vi "Main Responder.vi"(11 "CIFPluginManager in":refnum<class "CIFPluginManager.lvclass">) -> (0 "error out":errorcluster, 3 "Plugin Manager out":refnum<class "CIFPluginManager.lvclass">)   [LabVIEW 2021, in "CIFPluginManager.lvclass"]
uses:
  CIFPluginManager.lvclass
  gRPC/CIF_Manager_server/RPC Messages/cif_manager_RegisterPluginResponse.ctl
  CIFPluginManager.lvclass/CIFPluginManager.ctl
  <vilib>/Utility/miscctls.llb/LVMapReplaceAction.ctl
  gRPC/CIF_Manager_server/RPC Messages/cif_common_Empty.ctl
  <vilib>/CIF Foundation/CIF Core/CIFUtilities/CIFLogs/Typedef/Message Type.ctl
  <vilib>/CIF Foundation/CIF Core/CIFPluginManager/gRPC/CIF_Manager_client/RPC Messages/cif_common_Empty.ctl
  gRPC/CIF_Manager_server/RPC Messages/cif_manager_UnregisterPluginLoaderResponse.ctl
  gRPC/CIF_Manager_server/RPC Messages/cif_manager_QueryPluginTypesResponse.ctl
  gRPC/CIF_Manager_server/RPC Messages/cif_manager_PluginType.ctl
  gRPC/CIF_Manager_server/RPC Messages/cif_common_ShortVersion.ctl
  gRPC/CIF_Manager_server/RPC Messages/cif_management_common_PluginMetadata.ctl
  gRPC/CIF_Manager_server/RPC Messages/cif_manager_QueryAllChannelsResponse.ctl
  gRPC/CIF_Manager_server/RPC Messages/cif_management_common_Channels.ctl
  gRPC/CIF_Manager_server/RPC Messages/cif_management_common_Channel.ctl
  gRPC/CIF_Manager_server/RPC Messages/cif_management_common_ChannelDirection.ctl
  gRPC/CIF_Manager_server/RPC Messages/cif_management_common_ChannelPattern.ctl
  gRPC/CIF_Manager_server/RPC Messages/cif_manager_PingResponse.ctl
  gRPC/CIF_Manager_server/RPC Messages/cif_common_Status.ctl
  gRPC/CIF_Manager_server/RPC Messages/cif_manager_QueryErrorsResponse.ctl
  gRPC/CIF_Manager_server/RPC Messages/cif_manager_ErrorInfoList.ctl
  gRPC/CIF_Manager_server/RPC Messages/cif_manager_ErrorInfo.ctl
  gRPC/CIF_Manager_server/RPC Messages/cif_manager_QueryConfigResponse.ctl
  gRPC/CIF_Manager_server/RPC Messages/cif_manager_FileData.ctl
  gRPC/CIF_Manager_server/RPC Messages/cif_manager_QueryInfoResponse.ctl
  gRPC/CIF_Manager_server/RPC Messages/cif_manager_ResetErrorIndexResponse.ctl
  gRPC/CIF_Manager_server/RPC Messages/cif_manager_ResetConfigIndexResponse.ctl
  gRPC/CIF_Manager_server/RPC Messages/cif_manager_ResetInfoIndexResponse.ctl
  gRPC/CIF_Manager_server/RPC Messages/cif_manager_QueryPluginInfoResponse.ctl
  gRPC/CIF_Manager_server/RPC Messages/cif_manager_PluginInfoArray.ctl
  gRPC/CIF_Manager_server/RPC Messages/cif_manager_PluginInfo.ctl
  gRPC/CIF_Manager_server/RPC Messages/cif_management_common_PluginStatusData.ctl
  gRPC/CIF_Manager_server/RPC Messages/cif_management_common_PluginStatusData_PluginState.ctl
  gRPC/CIF_Manager_server/RPC Messages/cif_management_common_TimingStatistics.ctl
  gRPC/CIF_Manager_server/RPC Messages/cif_common_TimingStats.ctl
  gRPC/CIF_Manager_server/RPC Messages/cif_management_common_FifoStatistics.ctl
  gRPC/CIF_Manager_server/RPC Messages/cif_management_common_Error.ctl
  gRPC/CIF_Manager_server/RPC Messages/cif_management_common_MonitorDoubles.ctl
  gRPC/CIF_Manager_server/RPC Messages/cif_management_common_MonitorU64.ctl
  gRPC/CIF_Manager_server/RPC Messages/cif_management_common_MonitorI64.ctl
  gRPC/CIF_Manager_server/RPC Messages/cif_management_common_LoaderInfo.ctl
  gRPC/CIF_Manager_server/RPC Messages/cif_management_common_LoaderType.ctl
  gRPC/CIF_Manager_server/RPC Messages/cif_manager_QueryPluginResponse.ctl
  <vilib>/CIF Foundation/CIF Core/CIFCore/Common/Typedef/Errors.ctl
  gRPC/CIF_Manager_server/RPC Messages/cif_manager_QueryClockStatusResponse.ctl
  gRPC/CIF_Manager_server/RPC Messages/cif_manager_ClockStatusArray.ctl
  gRPC/CIF_Manager_server/RPC Messages/cif_manager_ClockStatus.ctl
  gRPC/CIF_Manager_server/RPC Messages/cif_manager_ClockConversion.ctl
  gRPC/CIF_Manager_server/RPC Messages/cif_manager_TimePair.ctl
  gRPC/CIF_Manager_server/RPC Messages/cif_manager_UpdateClockResponse.ctl
  <vilib>/CIF Foundation/CIF Utilities/Time/Typedef/Timestamp Pair.ctl
  gRPC/CIF_Manager_server/RPC Messages/cif_manager_CreateOrchResponse.ctl
  gRPC/CIF_Manager_server/RPC Messages/cif_manager_DestroyPluginLoaderResponse.ctl
  gRPC/CIF_Manager_server/RPC Messages/Get cif_manager_RegisterPluginRequest.vi
  gRPC/CIF_Manager_server/RPC Messages/Set cif_manager_RegisterPluginResponse.vi
  gRPC/CIF_Manager_server/RPC Messages/Get cif_manager_RegisterPluginLoaderRequest.vi
  gRPC/CIF_Manager_server/RPC Messages/Set cif_manager_RegisterPluginLoaderResponse.vi
  gRPC/CIF_Manager_server/RPC Messages/Get cif_manager_UnregisterPluginRequest.vi
  gRPC/CIF_Manager_server/RPC Messages/Set cif_manager_UnregisterPluginResponse.vi
  gRPC/CIF_Manager_server/RPC Messages/Get cif_manager_UnregisterPluginLoaderRequest.vi
  gRPC/CIF_Manager_server/RPC Messages/Set cif_manager_UnregisterPluginLoaderResponse.vi
  gRPC/CIF_Manager_server/RPC Messages/Get cif_manager_QueryPluginTypesRequest.vi
  gRPC/CIF_Manager_server/RPC Messages/Set cif_manager_QueryPluginTypesResponse.vi
  gRPC/CIF_Manager_server/RPC Messages/Get cif_manager_QueryAllChannelsRequest.vi
  gRPC/CIF_Manager_server/RPC Messages/Set cif_manager_QueryAllChannelsResponse.vi
  gRPC/CIF_Manager_server/RPC Messages/Get cif_manager_DestroyRequest.vi
  gRPC/CIF_Manager_server/RPC Messages/Set cif_manager_DestroyResponse.vi
  gRPC/CIF_Manager_server/RPC Messages/Get cif_manager_PingRequest.vi
  gRPC/CIF_Manager_server/RPC Messages/Set cif_manager_PingResponse.vi
  gRPC/CIF_Manager_server/RPC Messages/Get cif_manager_QueryErrorsRequest.vi
  gRPC/CIF_Manager_server/RPC Messages/Set cif_manager_QueryErrorsResponse.vi
  gRPC/CIF_Manager_server/RPC Messages/Get cif_manager_QueryConfigRequest.vi
  gRPC/CIF_Manager_server/RPC Messages/Set cif_manager_QueryConfigResponse.vi
  gRPC/CIF_Manager_server/RPC Messages/Get cif_manager_QueryInfoRequest.vi
  gRPC/CIF_Manager_server/RPC Messages/Set cif_manager_QueryInfoResponse.vi
  gRPC/CIF_Manager_server/RPC Messages/Get cif_manager_ResetErrorIndexRequest.vi
  gRPC/CIF_Manager_server/RPC Messages/Set cif_manager_ResetErrorIndexResponse.vi
  gRPC/CIF_Manager_server/RPC Messages/Get cif_manager_ResetConfigIndexRequest.vi
  gRPC/CIF_Manager_server/RPC Messages/Set cif_manager_ResetConfigIndexResponse.vi
  gRPC/CIF_Manager_server/RPC Messages/Get cif_manager_ResetInfoIndexRequest.vi
  gRPC/CIF_Manager_server/RPC Messages/Set cif_manager_ResetInfoIndexResponse.vi
  gRPC/CIF_Manager_server/RPC Messages/Get cif_manager_QueryPluginInfoRequest.vi
  gRPC/CIF_Manager_server/RPC Messages/Set cif_manager_QueryPluginInfoResponse.vi
  gRPC/CIF_Manager_server/RPC Messages/Get cif_manager_QueryPluginRequest.vi
  gRPC/CIF_Manager_server/RPC Messages/Set cif_manager_QueryPluginResponse.vi
  <vilib>/CIF Foundation/CIF Utilities/Errors/Append Error Location.vi
  gRPC/CIF_Manager_server/RPC Messages/Get cif_manager_QueryClockStatusRequest.vi
  gRPC/CIF_Manager_server/RPC Messages/Set cif_manager_QueryClockStatusResponse.vi
  gRPC/CIF_Manager_server/RPC Messages/Get cif_manager_UpdateClockRequest.vi
  gRPC/CIF_Manager_server/RPC Messages/Set cif_manager_UpdateClockResponse.vi
  <vilib>/CIF Foundation/CIF Utilities/Time/SubVIs/Weighted Moving Average for Slope.vi
  <vilib>/CIF Foundation/CIF Utilities/DataTypes/Utilities/Valid Number.vi
  gRPC/CIF_Manager_server/RPC Messages/Get cif_manager_CreateOrchRequest.vi
  gRPC/CIF_Manager_server/RPC Messages/Set cif_manager_CreateOrchResponse.vi
  gRPC/CIF_Manager_server/RPC Messages/Get cif_manager_DestroyPluginLoaderRequest.vi
  gRPC/CIF_Manager_server/RPC Messages/Set cif_manager_DestroyPluginLoaderResponse.vi
  gRPC/CIF_Manager_server/RPC Messages/Get cif_manager_RegisterPluginRequest.vi/2ed25e12-861d-4677-8ead-ace2906b2041.vi
  gRPC/CIF_Manager_server/RPC Messages/FlatToRichcif_manager_RegisterPluginRequest.vi
  gRPC/CIF_Manager_server/RPC Messages/Set cif_manager_RegisterPluginResponse.vi/dcc74a39-081a-4bdd-860b-8ed792803c96.vi
  gRPC/CIF_Manager_server/RPC Messages/RichToFlatcif_manager_RegisterPluginResponse.vi
  gRPC/CIF_Manager_server/RPC Messages/Get cif_manager_RegisterPluginLoaderRequest.vi/2ed25e12-861d-4677-8ead-ace2906b2041.vi
  gRPC/CIF_Manager_server/RPC Messages/FlatToRichcif_manager_RegisterPluginLoaderRequest.vi
  gRPC/CIF_Manager_server/RPC Messages/Set cif_manager_RegisterPluginLoaderResponse.vi/dcc74a39-081a-4bdd-860b-8ed792803c96.vi
  gRPC/CIF_Manager_server/RPC Messages/RichToFlatcif_manager_RegisterPluginLoaderResponse.vi
  gRPC/CIF_Manager_server/RPC Messages/Get cif_manager_UnregisterPluginRequest.vi/2ed25e12-861d-4677-8ead-ace2906b2041.vi
  gRPC/CIF_Manager_server/RPC Messages/FlatToRichcif_manager_UnregisterPluginRequest.vi
  gRPC/CIF_Manager_server/RPC Messages/Set cif_manager_UnregisterPluginResponse.vi/dcc74a39-081a-4bdd-860b-8ed792803c96.vi
  gRPC/CIF_Manager_server/RPC Messages/RichToFlatcif_manager_UnregisterPluginResponse.vi
  gRPC/CIF_Manager_server/RPC Messages/Get cif_manager_UnregisterPluginLoaderRequest.vi/2ed25e12-861d-4677-8ead-ace2906b2041.vi
  gRPC/CIF_Manager_server/RPC Messages/FlatToRichcif_manager_UnregisterPluginLoaderRequest.vi
  gRPC/CIF_Manager_server/RPC Messages/Set cif_manager_UnregisterPluginLoaderResponse.vi/dcc74a39-081a-4bdd-860b-8ed792803c96.vi
  gRPC/CIF_Manager_server/RPC Messages/RichToFlatcif_manager_UnregisterPluginLoaderResponse.vi
  gRPC/CIF_Manager_server/RPC Messages/Get cif_manager_QueryPluginTypesRequest.vi/2ed25e12-861d-4677-8ead-ace2906b2041.vi
  gRPC/CIF_Manager_server/RPC Messages/FlatToRichcif_manager_QueryPluginTypesRequest.vi
  gRPC/CIF_Manager_server/RPC Messages/Set cif_manager_QueryPluginTypesResponse.vi/dcc74a39-081a-4bdd-860b-8ed792803c96.vi
  gRPC/CIF_Manager_server/RPC Messages/RichToFlatcif_manager_QueryPluginTypesResponse.vi
  gRPC/CIF_Manager_server/RPC Messages/Get cif_manager_QueryAllChannelsRequest.vi/2ed25e12-861d-4677-8ead-ace2906b2041.vi
  gRPC/CIF_Manager_server/RPC Messages/FlatToRichcif_manager_QueryAllChannelsRequest.vi
  gRPC/CIF_Manager_server/RPC Messages/Set cif_manager_QueryAllChannelsResponse.vi/dcc74a39-081a-4bdd-860b-8ed792803c96.vi
  gRPC/CIF_Manager_server/RPC Messages/RichToFlatcif_manager_QueryAllChannelsResponse.vi
  gRPC/CIF_Manager_server/RPC Messages/Get cif_manager_DestroyRequest.vi/2ed25e12-861d-4677-8ead-ace2906b2041.vi
  gRPC/CIF_Manager_server/RPC Messages/FlatToRichcif_manager_DestroyRequest.vi
  gRPC/CIF_Manager_server/RPC Messages/Set cif_manager_DestroyResponse.vi/dcc74a39-081a-4bdd-860b-8ed792803c96.vi
  gRPC/CIF_Manager_server/RPC Messages/RichToFlatcif_manager_DestroyResponse.vi
  gRPC/CIF_Manager_server/RPC Messages/Get cif_manager_PingRequest.vi/2ed25e12-861d-4677-8ead-ace2906b2041.vi
  gRPC/CIF_Manager_server/RPC Messages/FlatToRichcif_manager_PingRequest.vi
  gRPC/CIF_Manager_server/RPC Messages/Set cif_manager_PingResponse.vi/dcc74a39-081a-4bdd-860b-8ed792803c96.vi
  gRPC/CIF_Manager_server/RPC Messages/RichToFlatcif_manager_PingResponse.vi
  gRPC/CIF_Manager_server/RPC Messages/Get cif_manager_QueryErrorsRequest.vi/2ed25e12-861d-4677-8ead-ace2906b2041.vi
  gRPC/CIF_Manager_server/RPC Messages/FlatToRichcif_manager_QueryErrorsRequest.vi
  gRPC/CIF_Manager_server/RPC Messages/Set cif_manager_QueryErrorsResponse.vi/dcc74a39-081a-4bdd-860b-8ed792803c96.vi
  gRPC/CIF_Manager_server/RPC Messages/RichToFlatcif_manager_QueryErrorsResponse.vi
  gRPC/CIF_Manager_server/RPC Messages/Get cif_manager_QueryConfigRequest.vi/2ed25e12-861d-4677-8ead-ace2906b2041.vi
  gRPC/CIF_Manager_server/RPC Messages/FlatToRichcif_manager_QueryConfigRequest.vi
  gRPC/CIF_Manager_server/RPC Messages/Set cif_manager_QueryConfigResponse.vi/dcc74a39-081a-4bdd-860b-8ed792803c96.vi
  gRPC/CIF_Manager_server/RPC Messages/RichToFlatcif_manager_QueryConfigResponse.vi
  gRPC/CIF_Manager_server/RPC Messages/Get cif_manager_QueryInfoRequest.vi/2ed25e12-861d-4677-8ead-ace2906b2041.vi
  gRPC/CIF_Manager_server/RPC Messages/FlatToRichcif_manager_QueryInfoRequest.vi
  gRPC/CIF_Manager_server/RPC Messages/Set cif_manager_QueryInfoResponse.vi/dcc74a39-081a-4bdd-860b-8ed792803c96.vi
  gRPC/CIF_Manager_server/RPC Messages/RichToFlatcif_manager_QueryInfoResponse.vi
  gRPC/CIF_Manager_server/RPC Messages/Get cif_manager_ResetErrorIndexRequest.vi/2ed25e12-861d-4677-8ead-ace2906b2041.vi
  gRPC/CIF_Manager_server/RPC Messages/FlatToRichcif_manager_ResetErrorIndexRequest.vi
  gRPC/CIF_Manager_server/RPC Messages/Set cif_manager_ResetErrorIndexResponse.vi/dcc74a39-081a-4bdd-860b-8ed792803c96.vi
  gRPC/CIF_Manager_server/RPC Messages/RichToFlatcif_manager_ResetErrorIndexResponse.vi
  gRPC/CIF_Manager_server/RPC Messages/Get cif_manager_ResetConfigIndexRequest.vi/2ed25e12-861d-4677-8ead-ace2906b2041.vi
  gRPC/CIF_Manager_server/RPC Messages/FlatToRichcif_manager_ResetConfigIndexRequest.vi
  gRPC/CIF_Manager_server/RPC Messages/Set cif_manager_ResetConfigIndexResponse.vi/dcc74a39-081a-4bdd-860b-8ed792803c96.vi
  gRPC/CIF_Manager_server/RPC Messages/RichToFlatcif_manager_ResetConfigIndexResponse.vi
  gRPC/CIF_Manager_server/RPC Messages/Get cif_manager_ResetInfoIndexRequest.vi/2ed25e12-861d-4677-8ead-ace2906b2041.vi
  gRPC/CIF_Manager_server/RPC Messages/FlatToRichcif_manager_ResetInfoIndexRequest.vi
  gRPC/CIF_Manager_server/RPC Messages/Set cif_manager_ResetInfoIndexResponse.vi/dcc74a39-081a-4bdd-860b-8ed792803c96.vi
  gRPC/CIF_Manager_server/RPC Messages/RichToFlatcif_manager_ResetInfoIndexResponse.vi
  gRPC/CIF_Manager_server/RPC Messages/Get cif_manager_QueryPluginInfoRequest.vi/2ed25e12-861d-4677-8ead-ace2906b2041.vi
  gRPC/CIF_Manager_server/RPC Messages/FlatToRichcif_manager_QueryPluginInfoRequest.vi
  gRPC/CIF_Manager_server/RPC Messages/Set cif_manager_QueryPluginInfoResponse.vi/dcc74a39-081a-4bdd-860b-8ed792803c96.vi
  gRPC/CIF_Manager_server/RPC Messages/RichToFlatcif_manager_QueryPluginInfoResponse.vi
  gRPC/CIF_Manager_server/RPC Messages/Get cif_manager_QueryPluginRequest.vi/2ed25e12-861d-4677-8ead-ace2906b2041.vi
  gRPC/CIF_Manager_server/RPC Messages/FlatToRichcif_manager_QueryPluginRequest.vi
  gRPC/CIF_Manager_server/RPC Messages/Set cif_manager_QueryPluginResponse.vi/dcc74a39-081a-4bdd-860b-8ed792803c96.vi
  gRPC/CIF_Manager_server/RPC Messages/RichToFlatcif_manager_QueryPluginResponse.vi
  gRPC/CIF_Manager_server/RPC Messages/Get cif_manager_QueryClockStatusRequest.vi/2ed25e12-861d-4677-8ead-ace2906b2041.vi
  gRPC/CIF_Manager_server/RPC Messages/FlatToRichcif_manager_QueryClockStatusRequest.vi
  gRPC/CIF_Manager_server/RPC Messages/Set cif_manager_QueryClockStatusResponse.vi/dcc74a39-081a-4bdd-860b-8ed792803c96.vi
  gRPC/CIF_Manager_server/RPC Messages/RichToFlatcif_manager_QueryClockStatusResponse.vi
  gRPC/CIF_Manager_server/RPC Messages/Get cif_manager_UpdateClockRequest.vi/2ed25e12-861d-4677-8ead-ace2906b2041.vi
  gRPC/CIF_Manager_server/RPC Messages/FlatToRichcif_manager_UpdateClockRequest.vi
  gRPC/CIF_Manager_server/RPC Messages/Set cif_manager_UpdateClockResponse.vi/dcc74a39-081a-4bdd-860b-8ed792803c96.vi
  gRPC/CIF_Manager_server/RPC Messages/RichToFlatcif_manager_UpdateClockResponse.vi
  <vilib>/Analysis/3filter.llb/Savitzky-Golay Filter.vi
  <vilib>/Analysis/3filter.llb/Savitzky-Golay Filter (DBL).vi
  gRPC/CIF_Manager_server/RPC Messages/Get cif_manager_CreateOrchRequest.vi/2ed25e12-861d-4677-8ead-ace2906b2041.vi
  gRPC/CIF_Manager_server/RPC Messages/FlatToRichcif_manager_CreateOrchRequest.vi
  gRPC/CIF_Manager_server/RPC Messages/Set cif_manager_CreateOrchResponse.vi/dcc74a39-081a-4bdd-860b-8ed792803c96.vi
  gRPC/CIF_Manager_server/RPC Messages/RichToFlatcif_manager_CreateOrchResponse.vi
  gRPC/CIF_Manager_server/RPC Messages/Get cif_manager_DestroyPluginLoaderRequest.vi/2ed25e12-861d-4677-8ead-ace2906b2041.vi
  gRPC/CIF_Manager_server/RPC Messages/FlatToRichcif_manager_DestroyPluginLoaderRequest.vi
  gRPC/CIF_Manager_server/RPC Messages/Set cif_manager_DestroyPluginLoaderResponse.vi/dcc74a39-081a-4bdd-860b-8ed792803c96.vi
  gRPC/CIF_Manager_server/RPC Messages/RichToFlatcif_manager_DestroyPluginLoaderResponse.vi
  <vilib>/gRPC/LabVIEW gRPC Library/Shared/TranslateGrpcError.vi
  gRPC/CIF_Manager_server/RPC Messages/FlatToRichcif_common_ShortVersion.vi
  gRPC/CIF_Manager_server/RPC Messages/FlatToRichcif_management_common_LoaderInfoFull.vi
  gRPC/CIF_Manager_server/RPC Messages/RichToFlatcif_manager_PluginType.vi
  gRPC/CIF_Manager_server/RPC Messages/FlatToRichcif_management_common_ChannelFilter.vi
  gRPC/CIF_Manager_server/RPC Messages/RichToFlatcif_management_common_Channels.vi
  gRPC/CIF_Manager_server/RPC Messages/RichToFlatcif_common_Status.vi
  gRPC/CIF_Manager_server/RPC Messages/FlatToRichcif_manager_QuerySettings.vi
  gRPC/CIF_Manager_server/RPC Messages/RichToFlatcif_manager_ErrorInfoList.vi
  gRPC/CIF_Manager_server/RPC Messages/RichToFlatcif_manager_FileData.vi
  gRPC/CIF_Manager_server/RPC Messages/RichToFlatcif_manager_PluginInfoArray.vi
  gRPC/CIF_Manager_server/RPC Messages/RichToFlatcif_manager_PluginInfo.vi
  gRPC/CIF_Manager_server/RPC Messages/RichToFlatcif_manager_ClockStatusArray.vi
  gRPC/CIF_Manager_server/RPC Messages/FlatToRichcif_manager_TimePair.vi
  gRPC/CIF_Manager_server/RPC Messages/RichToFlatcif_common_ShortVersion.vi
  gRPC/CIF_Manager_server/RPC Messages/RichToFlatcif_management_common_PluginMetadata.vi
  gRPC/CIF_Manager_server/RPC Messages/RichToFlatcif_management_common_Channel.vi
  gRPC/CIF_Manager_server/RPC Messages/RichToFlatcif_manager_ErrorInfo.vi
  gRPC/CIF_Manager_server/RPC Messages/RichToFlatcif_management_common_PluginStatusData.vi
  gRPC/CIF_Manager_server/RPC Messages/RichToFlatcif_management_common_LoaderInfo.vi
  gRPC/CIF_Manager_server/RPC Messages/RichToFlatcif_manager_ClockStatus.vi
  gRPC/CIF_Manager_server/RPC Messages/RichToFlatcif_management_common_TimingStatistics.vi
  gRPC/CIF_Manager_server/RPC Messages/RichToFlatcif_management_common_FifoStatistics.vi
  gRPC/CIF_Manager_server/RPC Messages/RichToFlatcif_management_common_Error.vi
  gRPC/CIF_Manager_server/RPC Messages/RichToFlatcif_management_common_MonitorDoubles.vi
  gRPC/CIF_Manager_server/RPC Messages/RichToFlatcif_management_common_MonitorU64.vi
  gRPC/CIF_Manager_server/RPC Messages/RichToFlatcif_management_common_MonitorI64.vi
  gRPC/CIF_Manager_server/RPC Messages/RichToFlatcif_manager_ClockConversion.vi
  gRPC/CIF_Manager_server/RPC Messages/RichToFlatcif_common_TimingStats.vi
  gRPC/CIF_Manager_server/RPC Messages/RichToFlatcif_manager_TimePair.vi
  <vilib>/gRPC/LabVIEW gRPC Library/Server API/Server/Get Server DLL Path.vi
  <vilib>/Utility/error.llb/Error Cluster From Error Code.vi
  <vilib>/gRPC/LabVIEW gRPC Library/Server API/Message Requests/Complete Call.vi
  <vilib>/Analysis/baseanly.llb/Std Deviation and Variance.vi
  <vilib>/Analysis/6fits.llb/Linear Fit.vi
  <vilib>/regexp/Match Regular Expression.xnode
  <vilib>/CIF Foundation/CIF Core/CIFUtilities/CIFLogs/CIFLogs.lvlib
  <vilib>/CIF Foundation/CIF Core/CIFPluginManager/gRPC/CIF_Manager_Client_Wrapper/CIFManagerClientWrapper.lvlib
  <vilib>/CIF Foundation/CIF Core/CIFPluginManager/gRPC/CIF_Manager_client/CIF_Manager_client.lvlib
  gRPC/CIF_Manager_server/RPC Service/Manager/Manager.lvclass
  <vilib>/CIF Foundation/CIF Utilities/Time/Time_CIF_U.lvlib
  <vilib>/CIF Foundation/CIF Core/CIFCore/Grpc/CIFCoreWrapper/CIFCoreWrapper.lvlib
  <vilib>/CIF Foundation/CIF Core/CIFUtilities/CIFConfigurationFile/CIF Configuration File.lvlib
  gRPC/CIF_Manager_server/CIF_Manager_server.lvlib
  CIFPluginLoader/gRPC/CIF_Plugin_Loader_Client_Wrapper/CIFPluginLoaderClientWrapper.lvlib
  <vilib>/CIF Foundation/CIF Core/CIFCore/Common/CIFCoreCommon.lvlib
  CIFUtilities/Scripting/Orchestration/Python/Python Orchestration.lvlib
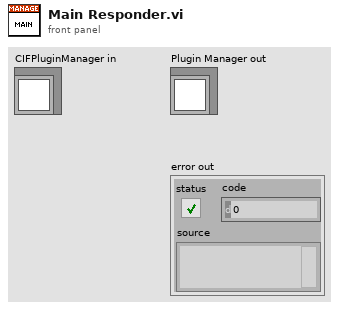
[diagram p1: front panel]
types:
  T1 = typedef "CIF_Manager_server.lvlib/cif_manager_RegisterPluginResponse.ctl" = cluster{"loader_name":string}
  T2 = typedef "LVMapReplaceAction.ctl" = enum32{"Modify Entry only if found", "Add or Modify Entry", "Delete Entry"}
  T3 = typedef "CIF_Manager_server.lvlib/cif_common_Empty.ctl" = cluster{"void":string}
  T4 = typedef "CIFLogs.lvlib/Message Type.ctl" = enum16{"Error", "Information", "Print Terminal", "Configuration"}
  T5 = typedef "CIF_Manager_client.lvlib/cif_common_Empty.ctl" = cluster{"void":string}
  T6 = typedef "CIF_Manager_server.lvlib/cif_manager_UnregisterPluginLoaderResponse.ctl" = cluster{"void":string}
  T7 = typedef "CIF_Manager_server.lvlib/cif_manager_QueryPluginTypesResponse.ctl" = cluster{"plugin_types":T8[]}
  T8 = typedef "CIF_Manager_server.lvlib/cif_manager_PluginType.ctl" = cluster{"plugin_type":string, "plugin_version":T9, "plugin_metadata":T10, "relative_path":string[]}
  T9 = typedef "CIF_Manager_server.lvlib/cif_common_ShortVersion.ctl" = cluster{"major":u32, "minor":u32, "fix":u32}
  T10 = typedef "CIF_Manager_server.lvlib/cif_management_common_PluginMetadata.ctl" = cluster{"description":string, "history":string, "author":string}
  T11 = typedef "CIF_Manager_server.lvlib/cif_manager_QueryAllChannelsResponse.ctl" = cluster{"channels":T12}
  T12 = typedef "CIF_Manager_server.lvlib/cif_management_common_Channels.ctl" = cluster{"channels":T13[]}
  T13 = typedef "CIF_Manager_server.lvlib/cif_management_common_Channel.ctl" = cluster{"name":string, "direction":T14, "type":string, "custom_config":u8[], "connected":bool, "connected_name":string, "forced":bool, "channel_pattern":T15}
  T14 = typedef "CIF_Manager_server.lvlib/cif_management_common_ChannelDirection.ctl" = enum32{"CHANNELDIRECTION_UNKNOWN", "CHANNELDIRECTION_PUBLISHER", "CHANNELDIRECTION_SUBSCRIBER"}
  T15 = typedef "CIF_Manager_server.lvlib/cif_management_common_ChannelPattern.ctl" = enum32{"CHANNELPATTERN_UNKNOWN", "CHANNELPATTERN_TAG", "CHANNELPATTERN_FIFO", "CHANNELPATTERN_MULTIFIFO", "CHANNELPATTERN_BACKPRESSUREFIFO"}
  T16 = typedef "CIF_Manager_server.lvlib/cif_manager_PingResponse.ctl" = cluster{"status":T17}
  T17 = typedef "CIF_Manager_server.lvlib/cif_common_Status.ctl" = cluster{"code":i32, "message":string}
  T18 = typedef "CIF_Manager_server.lvlib/cif_manager_QueryErrorsResponse.ctl" = cluster{"error_info_list":T19}
  T19 = typedef "CIF_Manager_server.lvlib/cif_manager_ErrorInfoList.ctl" = cluster{"error_info":T20[]}
  T20 = typedef "CIF_Manager_server.lvlib/cif_manager_ErrorInfo.ctl" = cluster{"error_status":bool, "error_code":i32, "plugin":string, "time":string, "message":string, "location":string}
  T21 = typedef "CIF_Manager_server.lvlib/cif_manager_QueryConfigResponse.ctl" = cluster{"file_data":T22}
  T22 = typedef "CIF_Manager_server.lvlib/cif_manager_FileData.ctl" = cluster{"data":string}
  T23 = typedef "CIF_Manager_server.lvlib/cif_manager_QueryInfoResponse.ctl" = cluster{"file_data":T22}
  T24 = typedef "CIF_Manager_server.lvlib/cif_manager_ResetErrorIndexResponse.ctl" = cluster{"status":T17}
  T25 = typedef "CIF_Manager_server.lvlib/cif_manager_ResetConfigIndexResponse.ctl" = cluster{"status":T17}
  T26 = typedef "CIF_Manager_server.lvlib/cif_manager_ResetInfoIndexResponse.ctl" = cluster{"status":T17}
  T27 = typedef "CIF_Manager_server.lvlib/cif_manager_QueryPluginInfoResponse.ctl" = cluster{"plugin_info_array":T28}
  T28 = typedef "CIF_Manager_server.lvlib/cif_manager_PluginInfoArray.ctl" = cluster{"plugin_info":T29[]}
  T29 = typedef "CIF_Manager_server.lvlib/cif_manager_PluginInfo.ctl" = cluster{"plugin_name":string, "plugin_type":string, "grpc_port":i32, "plugin_version":T9, "status":T30, "loader_info":T39}
  T30 = typedef "CIF_Manager_server.lvlib/cif_management_common_PluginStatusData.ctl" = cluster{"state":T31, "timing_statistics":T32, "fifo_statistics":T34, "error":T35, "monitor_doubles":T36, "monitor_u64s":T37, "monitor_i64s":T38}
  T31 = typedef "CIF_Manager_server.lvlib/cif_management_common_PluginStatusData_PluginState.ctl" = enum32{"PLUGINSTATE_UNKNOWN", "PLUGINSTATE_CREATING", "PLUGINSTATE_LISTENING", "PLUGINSTATE_RUNNING", "PLUGINSTATE_CLEANINGUP", "PLUGINSTATE_DESTROYING"}
  T32 = typedef "CIF_Manager_server.lvlib/cif_management_common_TimingStatistics.ctl" = cluster{"period":T33, "wake_error":T33, "execute":T33, "housekeep":T33, "idle":T33, "cleanup":T33, "custom_1":T33, "custom_2":T33}
  T33 = typedef "CIF_Manager_server.lvlib/cif_common_TimingStats.ctl" = cluster{"max":i64, "min":i64, "avg":dbl}
  T34 = typedef "CIF_Manager_server.lvlib/cif_management_common_FifoStatistics.ctl" = cluster{"from_t0":T33, "from_previous_plugin":T33, "output_error":T33}
  T35 = typedef "CIF_Manager_server.lvlib/cif_management_common_Error.ctl" = cluster{"status":bool, "code":i32}
  T36 = typedef "CIF_Manager_server.lvlib/cif_management_common_MonitorDoubles.ctl" = cluster{"double_1":dbl, "double_2":dbl, "double_3":dbl, "double_4":dbl}
  T37 = typedef "CIF_Manager_server.lvlib/cif_management_common_MonitorU64.ctl" = cluster{"u64_1":u64, "u64_2":u64, "u64_3":u64, "u64_4":u64}
  T38 = typedef "CIF_Manager_server.lvlib/cif_management_common_MonitorI64.ctl" = cluster{"i64_1":i64, "i64_2":i64, "i64_3":i64, "i64_4":i64}
  T39 = typedef "CIF_Manager_server.lvlib/cif_management_common_LoaderInfo.ctl" = cluster{"loader_type":T40, "loader_name":string}
  T40 = typedef "CIF_Manager_server.lvlib/cif_management_common_LoaderType.ctl" = enum32{"LOADERTYPE_UNKNOWN", "LOADERTYPE_LABVIEW"}
  T41 = typedef "CIF_Manager_server.lvlib/cif_manager_QueryPluginResponse.ctl" = cluster{"plugin_info":T29, "status":T17}
  T42 = typedef "CIFCoreCommon.lvlib/Errors.ctl" = enum16{"Invalid Clock ID", "Long Sleep", "gRPC Server Not Found", "Config Parse", "Timestamp Wrap", "Delayed Execution", "Duplicate Channel", "Missing Channel", "Incorrect Type", "Flatten Error", "Unflatten Data", "Unique Name", "Plugin Not Found", "Plugin Type Not Found", "Plugin Version Not Found", "Manager Not Found", "Numerical Issue", "Time Jump", "Clock ID Match", "Channel Length", "Plugin Connection", "gRPC Server Connection", "PPL Name Match", "Build", "Config Log Parse", "Plugin Load", "UI Subpanel Load", "Python Name", "Invalid Name", "Unable to Change Ch Buffer", "Failed Kill", "Failed SysExec", "Function Not Implemented", "Load Timeout"}
  T43 = typedef "CIF_Manager_server.lvlib/cif_manager_QueryClockStatusResponse.ctl" = cluster{"clock_status_array":T44}
  T44 = typedef "CIF_Manager_server.lvlib/cif_manager_ClockStatusArray.ctl" = cluster{"clocks_status":T45[]}
  T45 = typedef "CIF_Manager_server.lvlib/cif_manager_ClockStatus.ctl" = cluster{"clock_conversion":T46, "error_mean":i64, "error_std_dev":i64}
  T46 = typedef "CIF_Manager_server.lvlib/cif_manager_ClockConversion.ctl" = cluster{"clock_id":u32, "last_reset":i64, "slope":dbl, "offset_pair":T47, "clock_name":string}
  T47 = typedef "CIF_Manager_server.lvlib/cif_manager_TimePair.ctl" = cluster{"system_time":i64, "external_time":i64}
  T48 = typedef "CIF_Manager_server.lvlib/cif_manager_UpdateClockResponse.ctl" = cluster{"status":T17}
  T49 = typedef "Time_CIF_U.lvlib/Timestamp Pair.ctl" = cluster{"System Time":i64, "External Time":i64}
  T50 = typedef "CIF_Manager_server.lvlib/cif_manager_CreateOrchResponse.ctl" = cluster{"orchestration_script":string, "status":T17}
  T51 = typedef "CIF_Manager_server.lvlib/cif_manager_DestroyPluginLoaderResponse.ctl" = cluster{"status":T17}
  T52 = typedef "grpc-lvsupport-release.lvlib/grpcId.ctl" = u64
  T53 = typedef "CIF_Manager_server.lvlib/cif_manager_RegisterPluginRequest.ctl" = cluster{"plugin_name":string, "grpc_port":i32, "plugin_version":T9}
  T54 = typedef "CIFPluginManager.lvclass/Plugin Management Data Map.ctl" = map{string, T55}
  T55 = typedef "CIFPluginManager.lvclass/Plugin Management Data.ctl" = cluster{"Unique Name":string, "Plugin Type":string, "gRPC Port":i32, "gRPC ID":T52, "Loader Type":T56, "Loader":string, "Version":T57, "Load Timestamp":i64, "Unload Timestamp":i64, "Unloading":bool, "Ready for removal":bool, "status":T30, "channels":T12}
  T56 = typedef "CIFPluginManager.lvclass/Loader Type.ctl" = enum16{"LabVIEW"}
  T57 = typedef "CIFCoreCommon.lvlib/Version.ctl" = cluster{"Major":i32, "Minor":i32, "Fix":i32, "Build":i32}
  T58 = typedef "CIF_Manager_server.lvlib/cif_manager_RegisterPluginLoaderRequest.ctl" = cluster{"loader_info":T59}
  T59 = typedef "CIF_Manager_server.lvlib/cif_management_common_LoaderInfoFull.ctl" = cluster{"loader_type":T40, "loader_name":string, "grpc_port":i32, "pid":u32}
  T60 = typedef "CIFPluginManager.lvclass/Loader Map.ctl" = map{string, T61}
  T61 = typedef "CIFPluginManager.lvclass/Loaders.ctl" = cluster{"Loader Type":T56, "grpc_port":i32, "pid":u32, "gRPC ID":T52, "Load Timestamp":i64, "Unloading":bool, "Ready for removal":bool, "Unload Timestamp":i64}
  T62 = typedef "CIF_Manager_server.lvlib/cif_manager_UnregisterPluginRequest.ctl" = cluster{"plugin_name":string, "unregister_channels":string[]}
  T63 = typedef "CIF_Manager_server.lvlib/cif_manager_UnregisterPluginLoaderRequest.ctl" = cluster{"loader_name":string}
  T64 = typedef "CIF_Manager_server.lvlib/cif_manager_QueryPluginTypesRequest.ctl" = cluster{"reload":bool}
  T65 = typedef "CIFPluginManager.lvclass/Discovered Plugin Map.ctl" = map{string, T66[]}
  T66 = typedef "CIFPluginManager.lvclass/Discovered Plugin.ctl" = cluster{"Filename":string, "Plugin Type":string, "Qualified name":string, "Version":T57, "Plugin Metadata":T67, "Loader Type":T56, "File Path":string, "Relative Path":string[]}
  T67 = typedef "CIFPluginManager.lvclass/Plugin Metadata.ctl" = cluster{"Description":string, "History":string, "Author":string}
  T68 = typedef "CIF_Manager_server.lvlib/cif_manager_QueryAllChannelsRequest.ctl" = cluster{"channel_filter":T69}
  T69 = typedef "CIF_Manager_server.lvlib/cif_management_common_ChannelFilter.ctl" = cluster{"name_regex":string, "direction":T14, "direction_filter":bool, "type_regex":string, "forced":bool, "forced_filter":bool}
  T70 = typedef "CIF_Manager_client.lvlib/cif_common_Status.ctl" = cluster{"code":i32, "message":string}
  T71 = typedef "CIF_Manager_server.lvlib/cif_manager_QueryErrorsRequest.ctl" = cluster{"query_settings":T72}
  T72 = typedef "CIF_Manager_server.lvlib/cif_manager_QuerySettings.ctl" = cluster{"query_all":bool}
  T73 = typedef "CIFLogs.lvlib/Error Message.ctl" = cluster{"error":bool, "code":i32, "Message":string, "Location":string, "Plugin":string, "Time":string}
  T74 = typedef "CIF_Manager_server.lvlib/cif_manager_QueryConfigRequest.ctl" = cluster{"query_settings":T72}
  T75 = typedef "CIF_Manager_server.lvlib/cif_manager_QueryInfoRequest.ctl" = cluster{"query_settings":T72}
  T76 = typedef "CIFLogs.lvlib/Log Info.ctl" = cluster{"size (bytes)":i64, "Last Timestamp":string}
  T77 = typedef "CIF_Manager_server.lvlib/cif_manager_QueryPluginRequest.ctl" = cluster{"plugin_name":string}
  T78 = typedef "Time_CIF_U.lvlib/Clock History Map.ctl" = map{u8, T79}
  T79 = typedef "Time_CIF_U.lvlib/Clock History.ctl" = cluster{"System Clock":i64[], "External Clock":i64[], "Last Reset Time":i64, "slope":dbl, "1/slope":dbl, "Offset Pair":T49, "Name":string}
  T80 = typedef "Time_CIF_U.lvlib/Clock Conversion.ctl" = cluster{"ClockID":u8, "Last Reset":i64, "Offset Pair":T49, "Slope":dbl, "1/Slope":dbl, "Name":string}
  T81 = typedef "Time_CIF_U.lvlib/Clock Error Statistics.ctl" = cluster{"mean":i64, "standard deviation":i64}
  T82 = typedef "CIF_Manager_server.lvlib/cif_manager_UpdateClockRequest.ctl" = cluster{"clock_id":u32, "timestamp_pair":T47, "reinit":bool, "clock_name":string}
  T83 = typedef "CIF_Manager_server.lvlib/cif_manager_CreateOrchRequest.ctl" = cluster{"start_timestamp":u64, "create_file":bool, "orchestration_language":T84, "filename":string, "default_ip":string}
  T84 = typedef "CIF_Manager_server.lvlib/cif_manager_OrchestrationLanguage.ctl" = enum32{"ORCHESTRATIONLANGUAGE_UNKNOWN", "ORCHESTRATIONLANGUAGE_PYTHON"}
  T85 = typedef "CIF_Manager_server.lvlib/cif_manager_DestroyPluginLoaderRequest.ctl" = cluster{"loader_name":string}
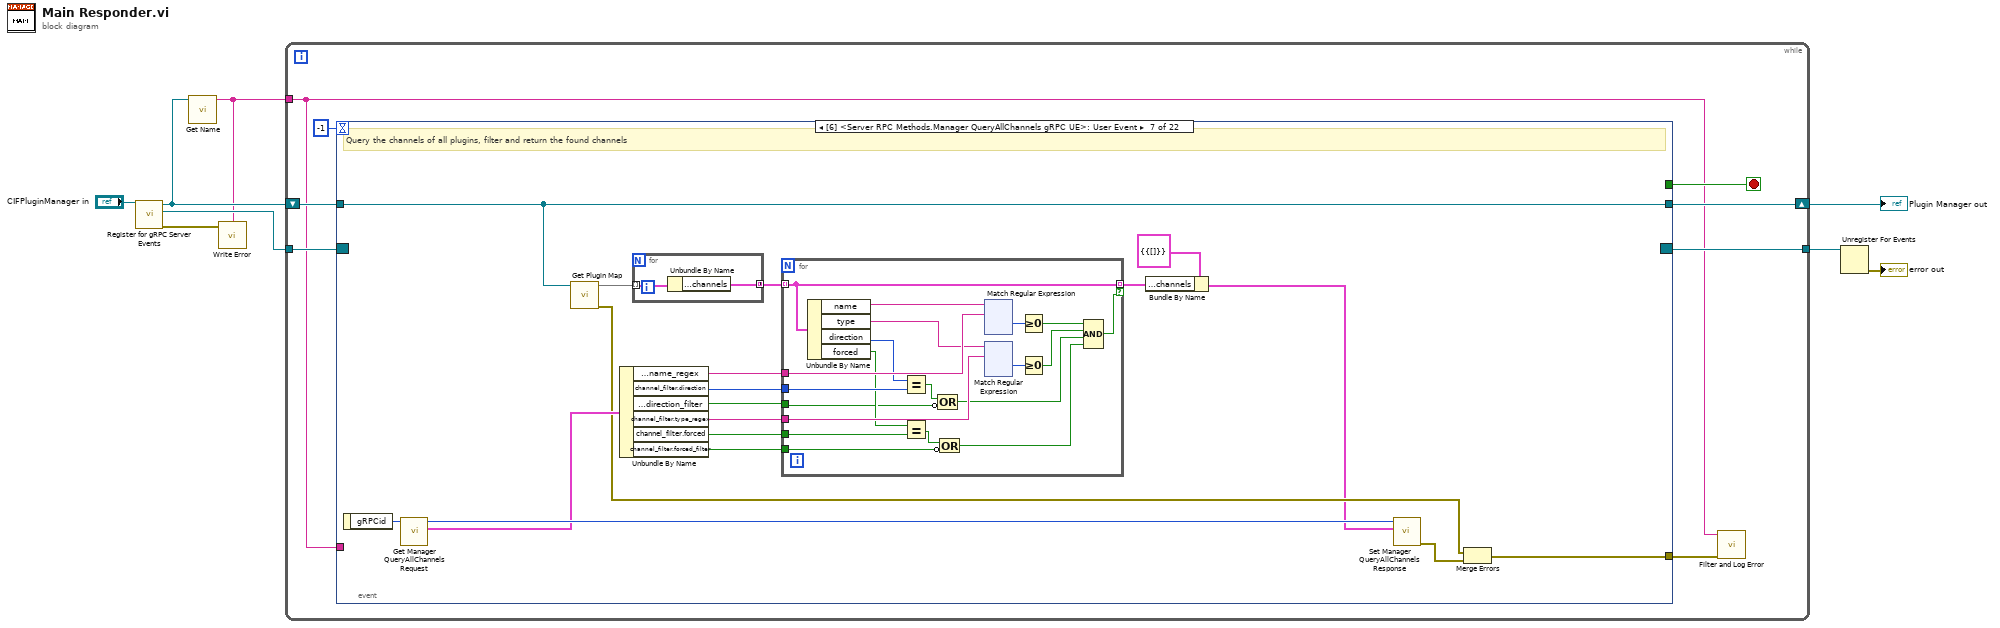
[diagram p0: block diagram]
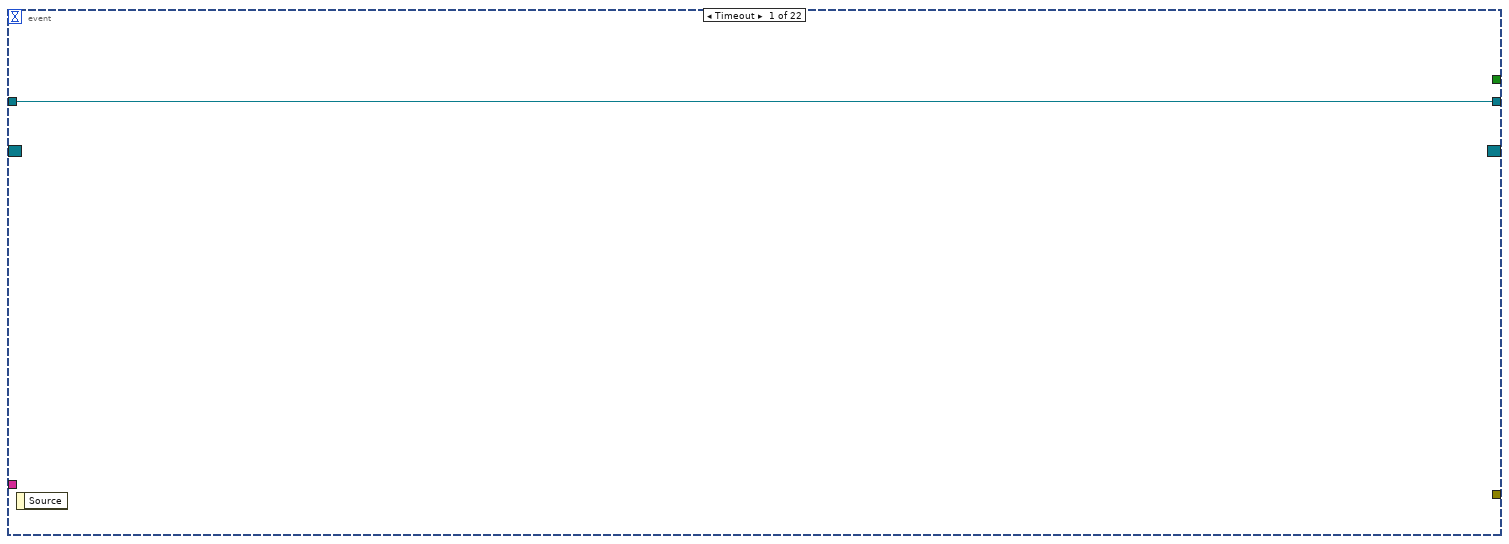
[diagram p2: hidden frame]
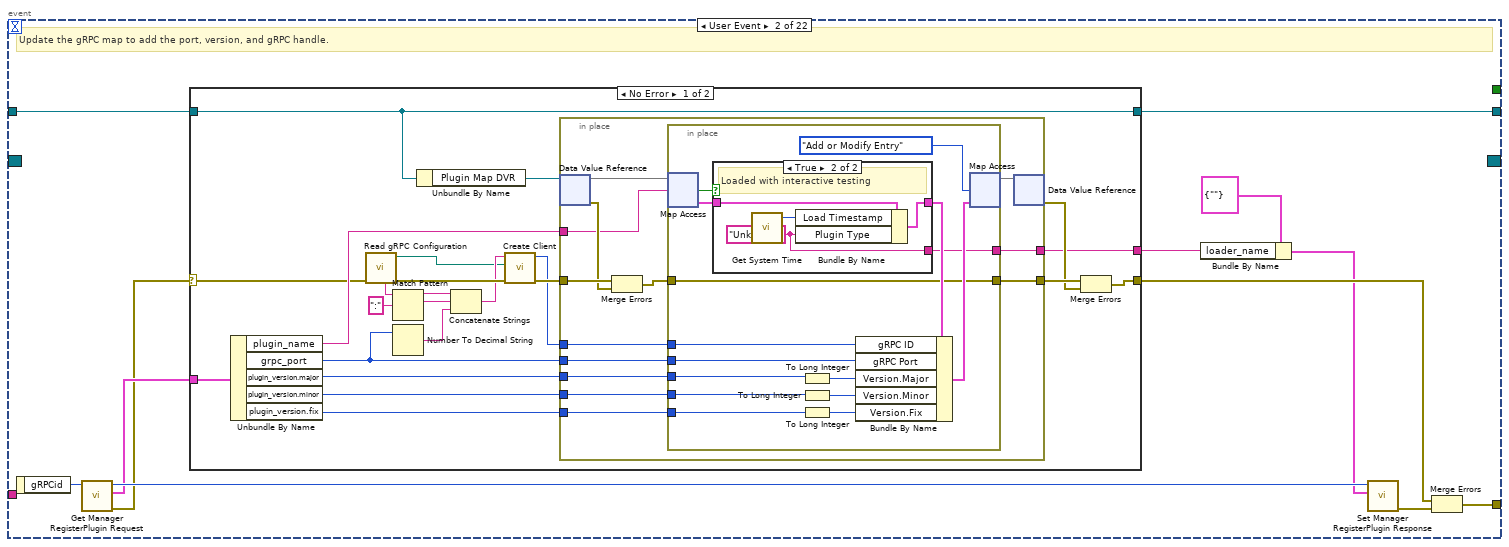
[diagram p3: hidden frame]
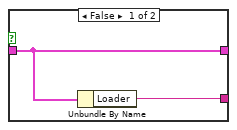
[diagram p4: hidden frame]
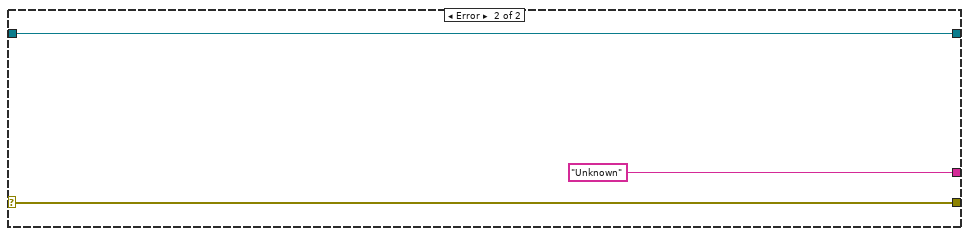
[diagram p5: hidden frame]
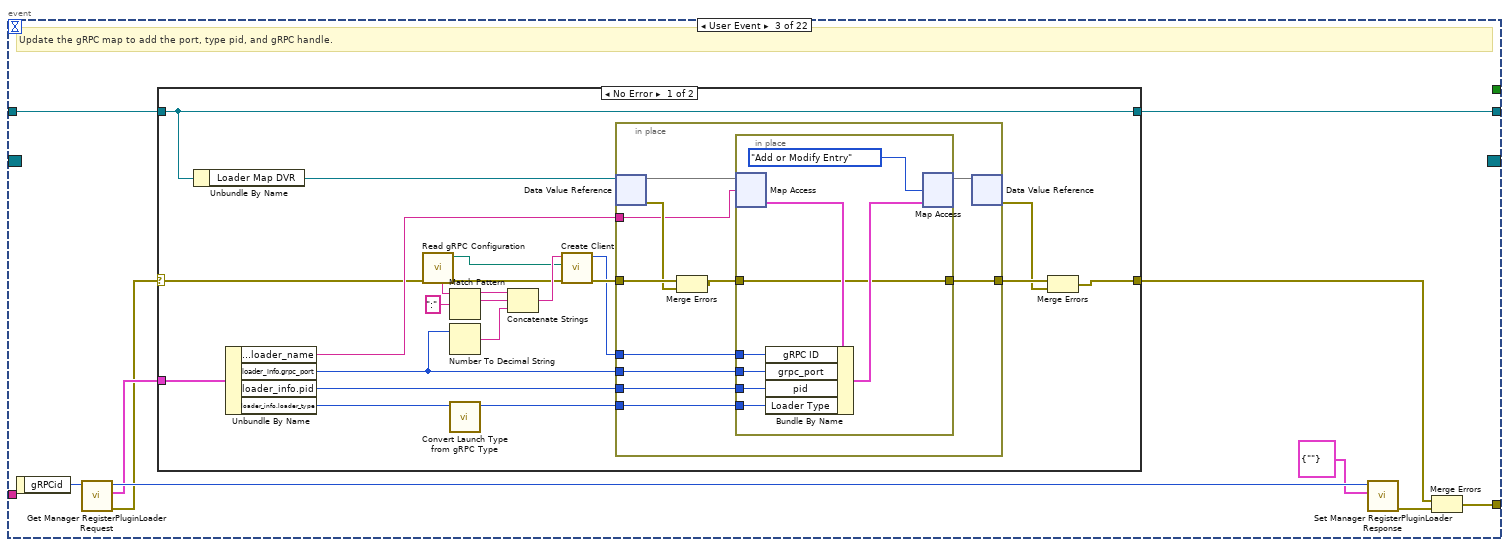
[diagram p6: hidden frame]
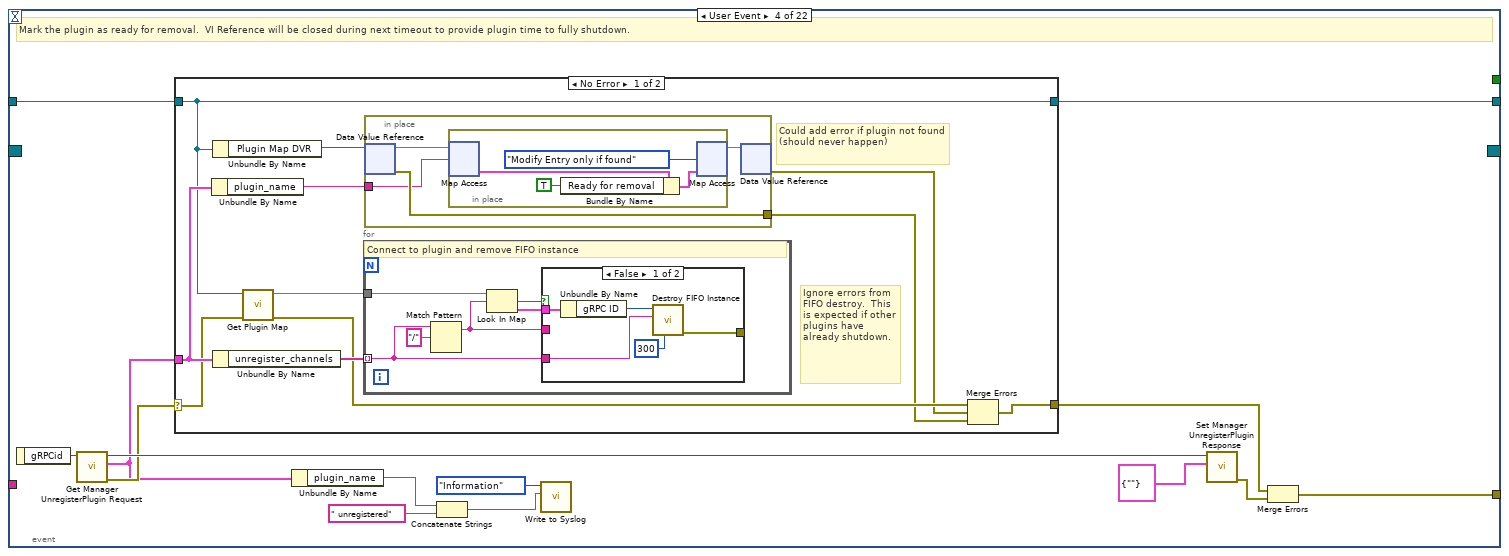
[diagram p8: hidden frame]
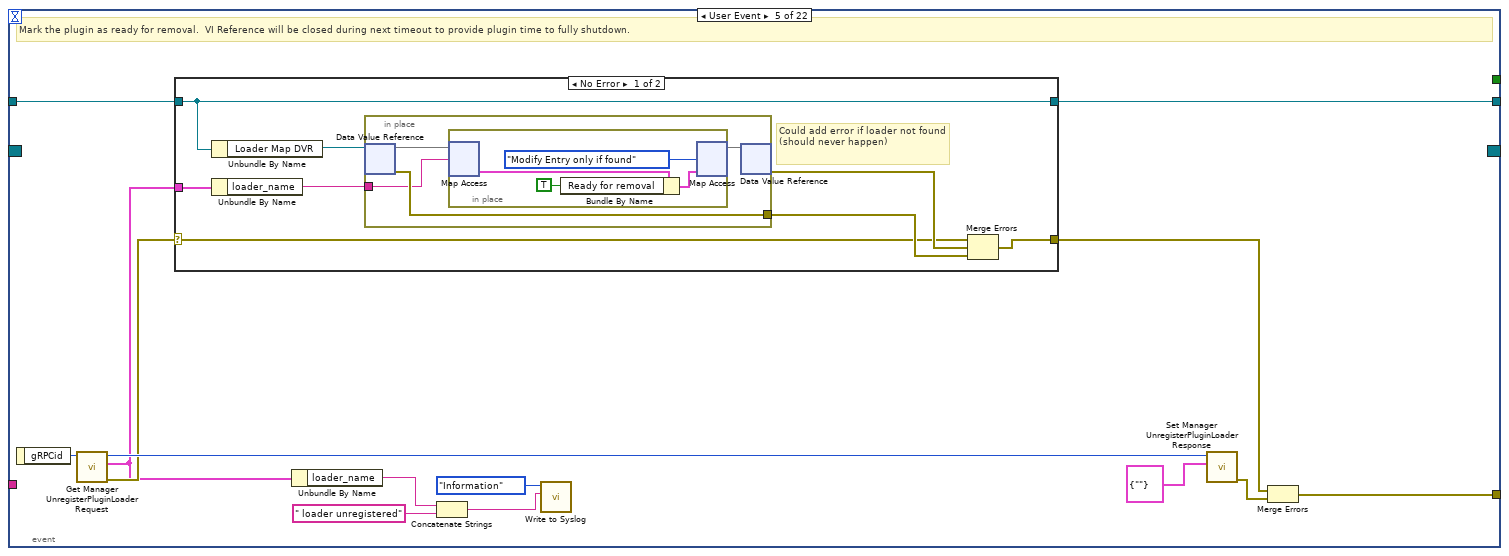
[diagram p11: hidden frame]
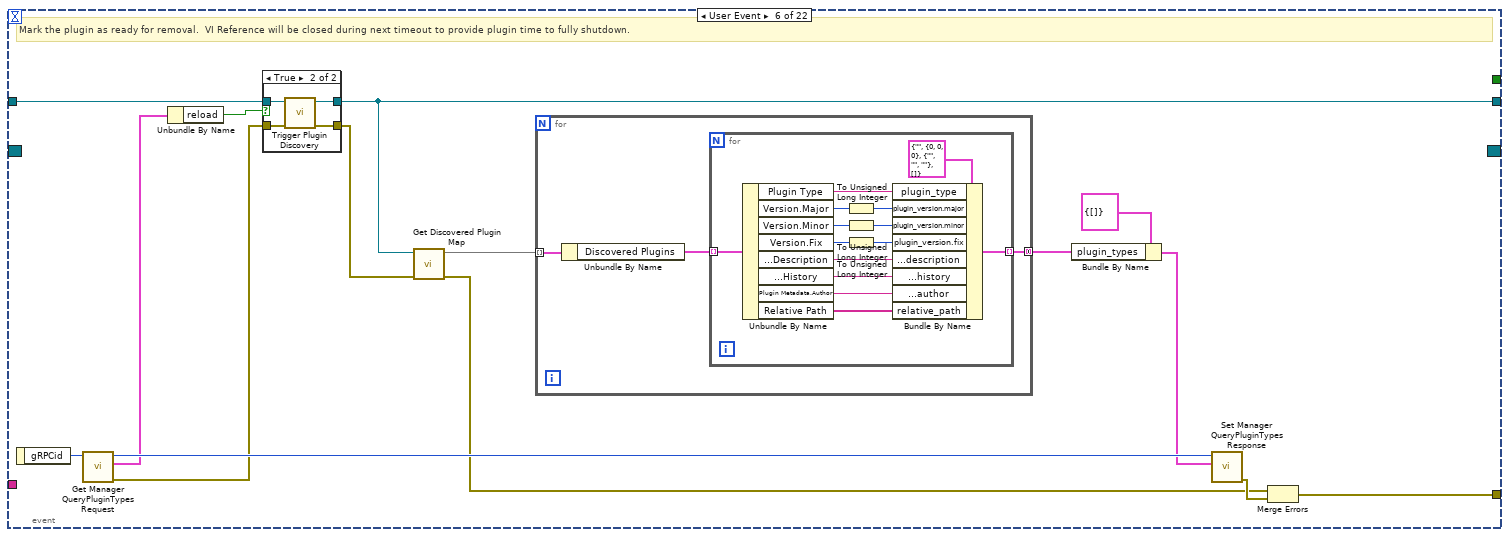
[diagram p13: hidden frame]
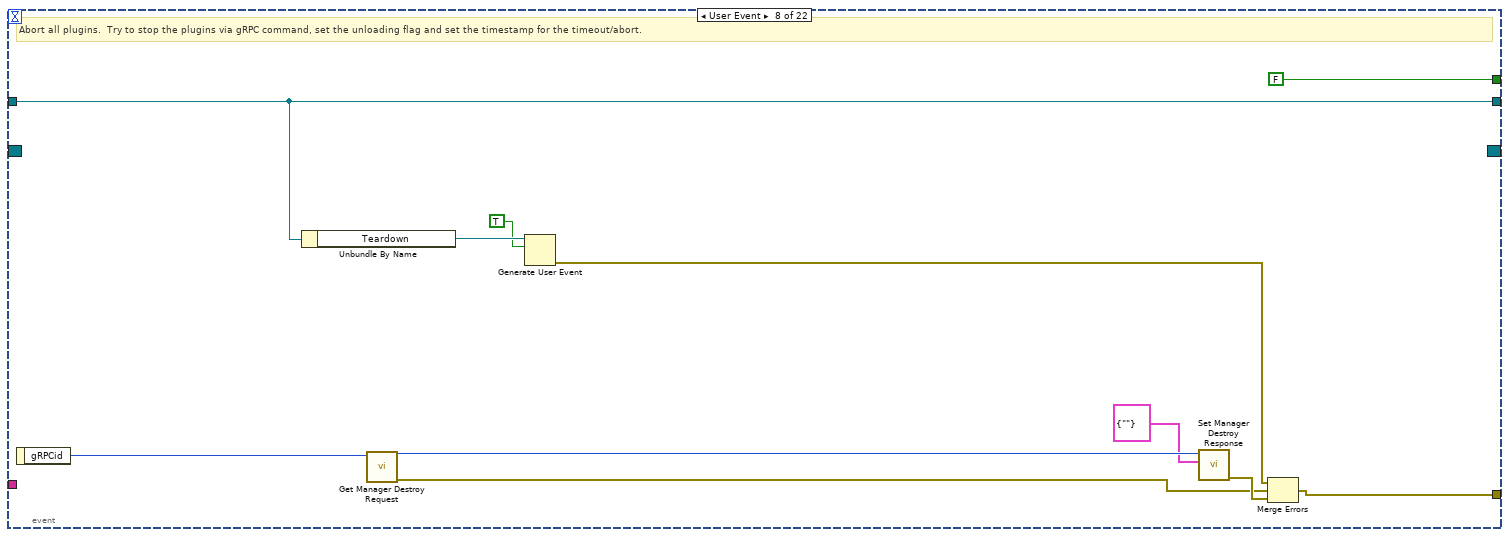
[diagram p15: hidden frame]
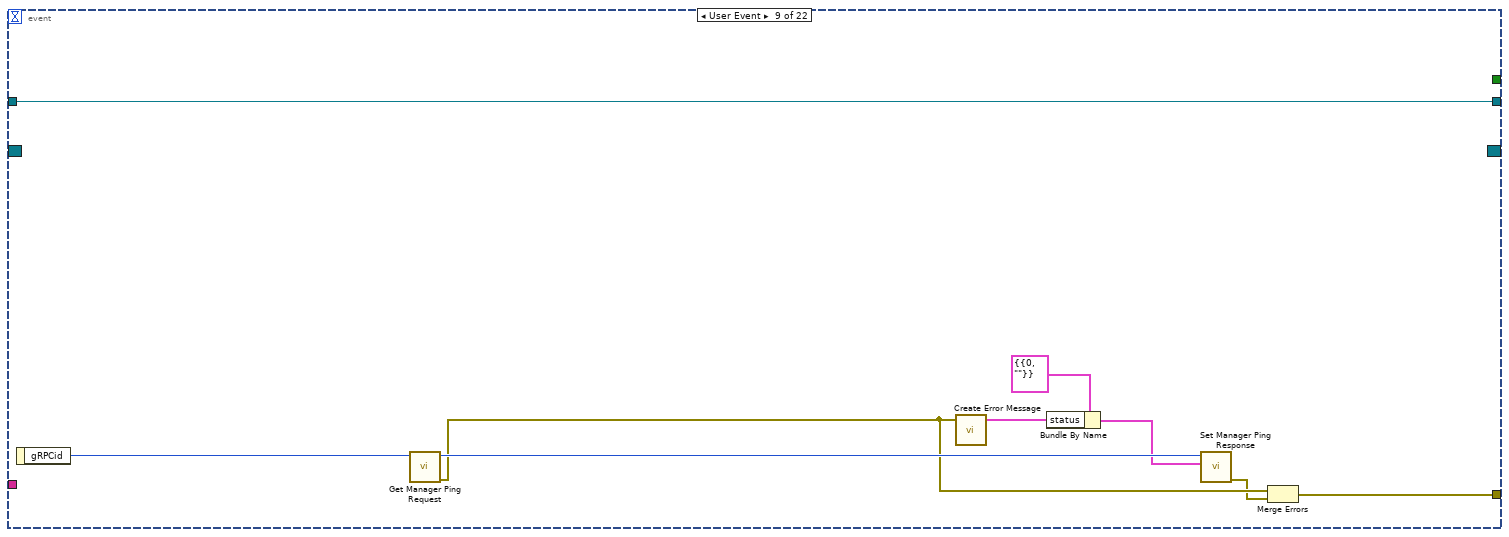
[diagram p16: hidden frame]
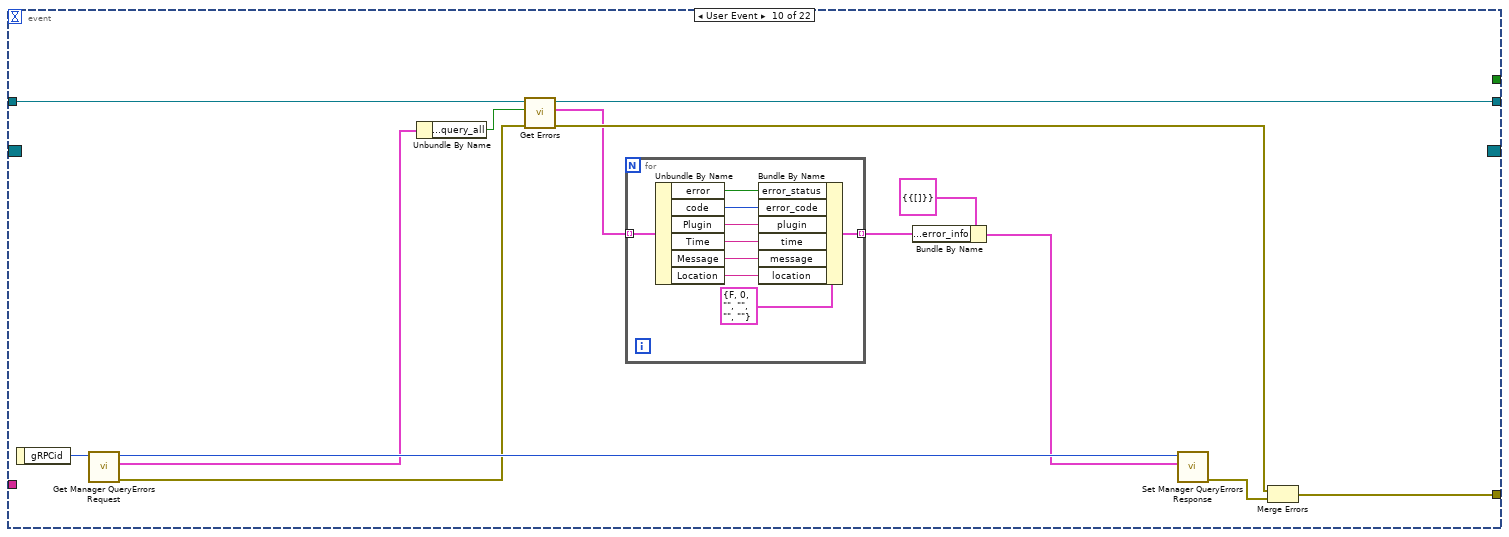
[diagram p17: hidden frame]
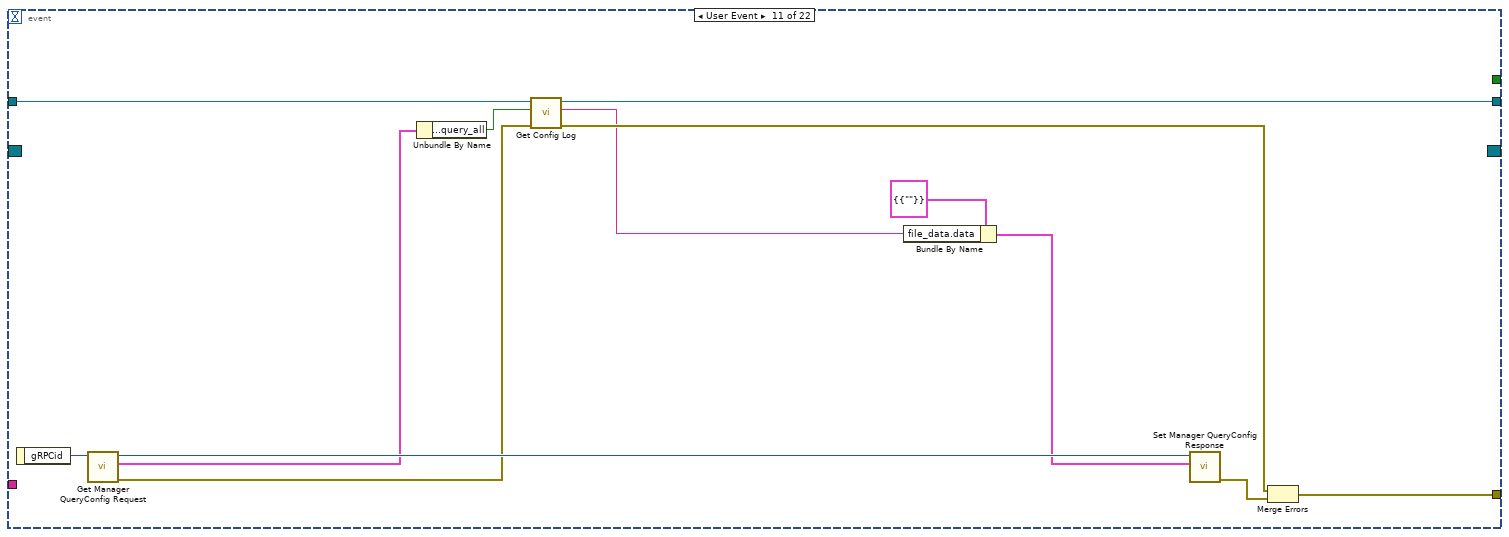
[diagram p18: hidden frame]
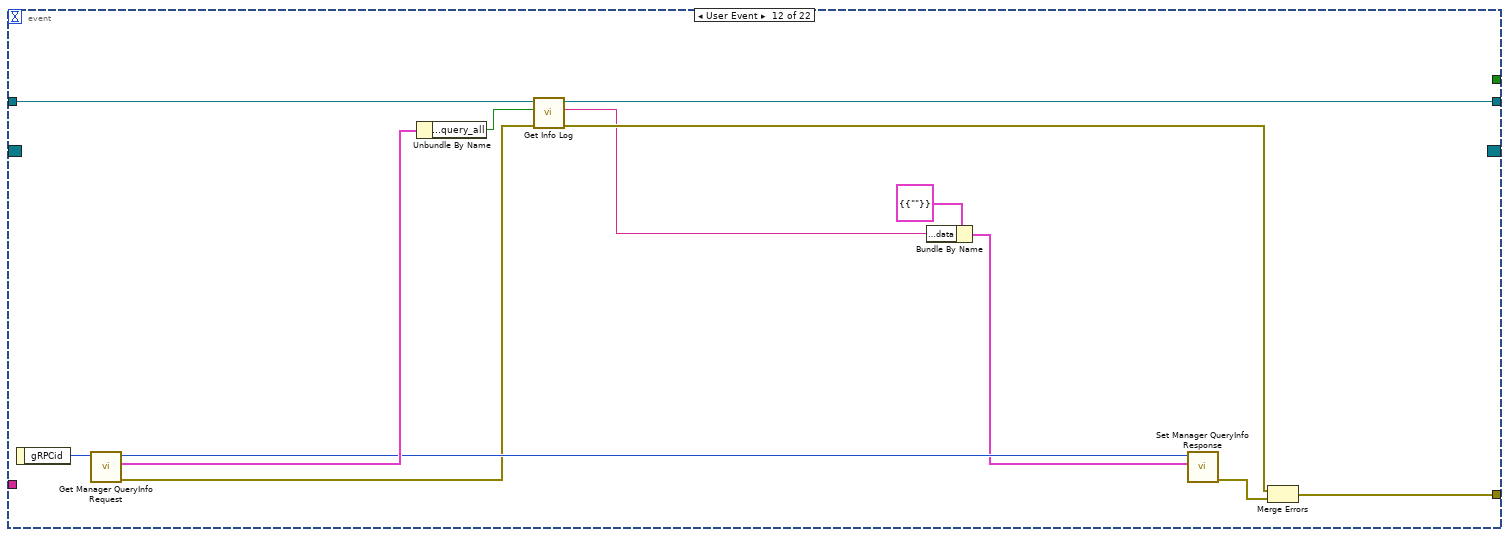
[diagram p19: hidden frame]
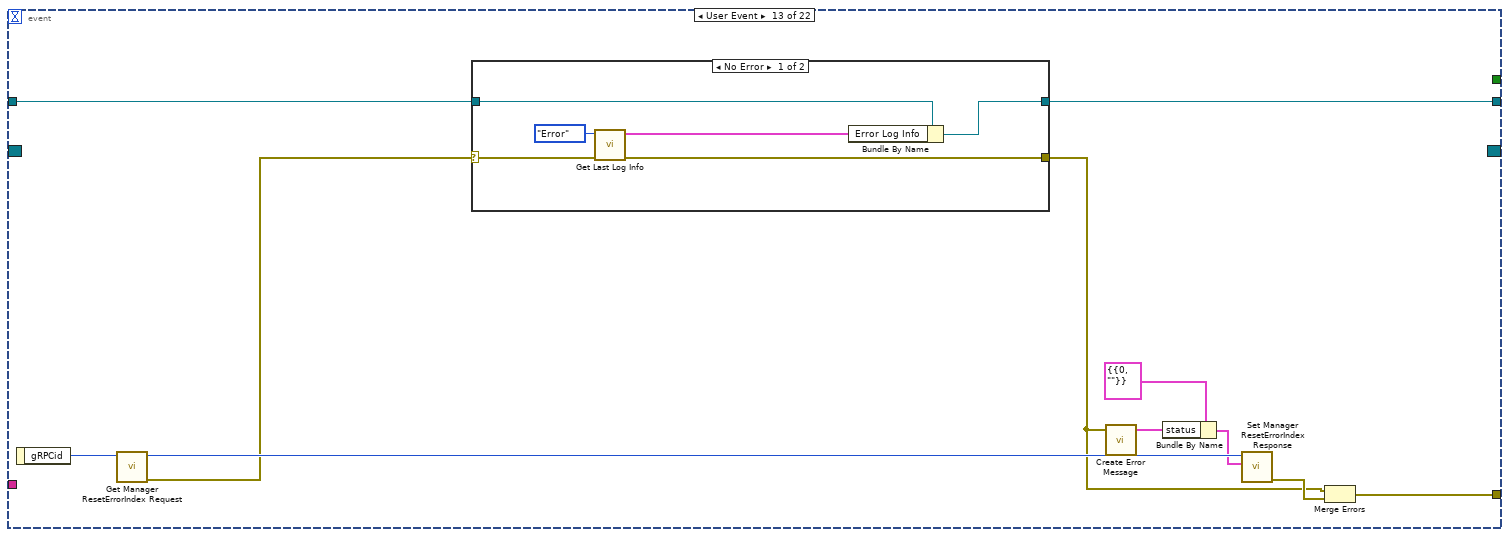
[diagram p20: hidden frame]
diagram:
  n1 = call "Register for gRPC Server Events.vi"("Plugin Manager in"="CIFPluginManager in") -> ("error out"=w8:errorcluster, "Event Registration Refnum"=w3:refnum<event-registration>, "Plugin Manager out"=w2:refnum<class "CIFPluginManager.lvclass">)  [unwired: 8 in]
  n2 = call "Get Name.vi"("CIFPluginManager in"=w2) -> ("Name"=w1:string)  [unwired: 10 in]
  n3 = call <vilib>:"Write Error.vi"("error in (no error)"=w8, "Plugin Name"=w1) -> ()  [unwired: 2 in, 1 out]
  n4 = while {
    tunnel: [w15] -> w6
    shift-right: [w14] -> w5
    shift-left: w2 -> [w16]
    tunnel: w3 -> [w11]
    tunnel: w1 -> [w9]
    stop <- w10 stop-if-true
    n5 = event shown="[6] <Server RPC Methods.Manager QueryAllChannels gRPC UE>: User Event" {
      selector: w11 -> [_ _ _ _ _ _ _ _ _ _ _ _ _ _ _ _ _ _ _ _ _ _]
      dyn-events: [_ _ _ _ _ _ _ _ _ _ _ _ _ _ _ _ _ _ _ _ _ _] -> w15
      timeout: -1 -> [_ _ _ _ _ _ _ _ _ _ _ _ _ _ _ _ _ _ _ _ _ _]
      tunnel: w16 -> [w17 w24 w94 w155 w201 w229 w263 w536 w547 w562 w583 w596 w607 w630 w646 w663 w692 w718 w748 w798 w824 w833]
      tunnel: [w17 w22 w92 w154 w200 w225 w263 w536 w547 w558 w580 w592 w606 w629 w644 w663 w692 w718 w748 w797 w824 w833] -> w14
      tunnel: [_ w29 w99 w156 w202 w235 w276 w543 w548 w566 w588 w601 w612 w631 w650 w669 w712 w726 w754 w802 w831 _] -> w13
      tunnel: [_ _ _ _ _ _ _ FALSE _ _ _ _ _ _ _ _ _ _ _ _ _ TRUE] -> w10
      tunnel: w9 -> [_ _ _ _ _ _ _ _ _ _ _ _ _ _ _ _ _ _ _ _ _ _]
      event Timeout {
        n6 = event-data() -> ()  [unwired: 1 in, 1 out]
      }
      event User Event {
        # "Update the gRPC map to add the port, version, and gRPC handle."
        n7 = event-data() -> ("gRPCid"=w27:T52)  [unwired: 1 in]
        n8 = call "Get Manager RegisterPlugin Request.vi"("gRPCid"=w27) -> ("error out"=w23:errorcluster, "Message Data"=w25:T53, "gRPCid out"=w28:T52)  [unwired: 8 in]
        n9 = case shown="No Error" w23 {
          selector: w23 -> [w36 w88]
          tunnel: w25 -> [w47 _]
          tunnel: w24 -> [w52 w89]
          tunnel: [w52 w89] -> w22
          tunnel: [w48 w88] -> w21
          tunnel: [w30 "Unknown" ("Loader")] -> w18
          frame No Error {
            n10 = Unbundle By Name(w47) -> ("plugin_name"=w46:string, "grpc_port"=w34:i32, "plugin_version.major"=w45:u32, "plugin_version.minor"=w44:u32, "plugin_version.fix"=w43:u32)
            n11 = call <vilib>:"Read gRPC Configuration.vi"("error in"=w36) -> ("error out"=w38:errorcluster, "Server Certificate File (.crt)"=w31:path, "Local Manager Address"=w39:string)  [unwired: 5 in, 3 out]
            n12 = Match Pattern(string=w39, regular expression=":") -> (before substring=w40:string, match substring=w41:string)  [unwired: 1 in, 2 out]
            n13 = Number To Decimal String(number=w34) -> (decimal integer string=w42:string)  [unwired: 1 in]
            n14 = Unbundle By Name(w52) -> ("Plugin Map DVR"=w51:refnum<data-value>)
            n15 = Concatenate Strings(w40, w41, w42) -> (w33:string)
            n16 = call <vilib>:"Create Client.vi"("error in"=w38, "Server Certificate File (.crt)"=w31, "address"=w33) -> ("error out"=w35:errorcluster, "gRPC ID Out"=w32:T52)  [unwired: 7 in]
            n17 = in-place {
              in-place-border: w35 -> [w63]
              in-place-border: [w65] -> w50
              in-place-border: w46 -> [w59]
              in-place-border: w34 -> [w58]
              in-place-border: w45 -> [w57]
              in-place-border: w44 -> [w56]
              in-place-border: w43 -> [w55]
              in-place-border: w32 -> [w54]
              in-place-border: [w53] -> w30
              n18 = in-place-dvr #1(w51) -> (w64:T54, w62:errorcluster)
              n19 = Merge Errors(w63, w62) -> (w61:errorcluster)
              n20 = in-place {
                in-place-border: w61 -> [w69]
                in-place-border: [w69] -> w65
                in-place-border: w58 -> [w73]
                in-place-border: w57 -> [w72]
                in-place-border: w56 -> [w71]
                in-place-border: w55 -> [w70]
                in-place-border: w54 -> [w68]
                in-place-border: [w66] -> w53
                n21 = in-place-map #2(w64, w59) -> (w67:T55, w75:bool)  [unwired: 1 in]
                n22 = case shown="True" w75 {
                  tunnel: w67 -> [w82 w86]
                  tunnel: [w82 w85] -> w74
                  tunnel: [w81 w83] -> w66
                  frame False {
                    n23 = Unbundle By Name(w82) -> ("Loader"=w81:string)
                  }
                  frame True {
                    w83 = "Unknown" ("Plugin Type")
                    # "Loaded with interactive testing"
                    n24 = call <vilib>:"Get System Time.vi"() -> ("Time (ns)"=w84:i64)  [unwired: 5 in]
                    n25 = Bundle By Name(cluster=w86, "Load Timestamp"=w84, "Plugin Type"=w83) -> (w85:T55)
                  }
                }
                n26 = To Long Integer(number=w72) -> (32bit integer=w78:i32)
                n27 = To Long Integer(number=w71) -> (32bit integer=w77:i32)
                n28 = To Long Integer(number=w70) -> (32bit integer=w76:i32)
                n29 = Bundle By Name(cluster=w74, "gRPC ID"=w68, "gRPC Port"=w73, "Version.Major"=w78, "Version.Minor"=w77, "Version.Fix"=w76) -> (w80:T55)
                n30 = in-place-map #2(w80, LVMapReplaceAction."Add or Modify Entry" ("action")) -> (w60:T54)  [unwired: 2 out]
              }
              n31 = in-place-dvr #1(w60) -> (w49:errorcluster)  [unwired: 1 out]
            }
            n32 = Merge Errors(w50, w49) -> (w48:errorcluster)
          }
          frame Error {
          }
        }
        n33 = Bundle By Name(cluster=T1 {"loader_name"=""} ("Message Data"), "loader_name"=w18) -> (w19:T1)
        n34 = call "Set Manager RegisterPlugin Response.vi"("Message Data"=w19, "gRPCid in"=w28) -> ("error out"=w26:errorcluster)  [unwired: 9 in]
        n35 = Merge Errors(w21, w26) -> (w29:errorcluster)
      }
      event User Event {
        # "Update the gRPC map to add the port, type pid, and gRPC handle."
        n36 = event-data() -> ("gRPCid"=w97:T52)  [unwired: 1 in]
        n37 = call "Get Manager RegisterPluginLoader Request.vi"("gRPCid"=w97) -> ("error out"=w93:errorcluster, "Message Data"=w95:T58, "gRPCid out"=w98:T52)  [unwired: 8 in]
        n38 = case shown="No Error" w93 {
          selector: w93 -> [w105 w141]
          tunnel: w95 -> [w116 _]
          tunnel: w94 -> [w121 w142]
          tunnel: [w121 w142] -> w92
          tunnel: [w117 w141] -> w91
          frame No Error {
            n39 = Unbundle By Name(w121) -> ("Loader Map DVR"=w120:refnum<data-value>)
            n40 = Unbundle By Name(w116) -> ("loader_info.loader_name"=w115:string, "loader_info.grpc_port"=w103:i32, "loader_info.pid"=w114:u32, "loader_info.loader_type"=w101:T40)
            n41 = call <vilib>:"Read gRPC Configuration.vi"("error in"=w105) -> ("error out"=w107:errorcluster, "Server Certificate File (.crt)"=w112:path, "Local Manager Address"=w108:string)  [unwired: 5 in, 3 out]
            n42 = Match Pattern(string=w108, regular expression=":") -> (before substring=w109:string, match substring=w110:string)  [unwired: 1 in, 2 out]
            n43 = Number To Decimal String(number=w103) -> (decimal integer string=w111:string)  [unwired: 1 in]
            n44 = call "Convert Launch Type from gRPC Type.vi"("Loader Type"=w101) -> ("Loader Type"=w100:T56)  [unwired: 9 in, 1 out]
            n45 = Concatenate Strings(w109, w110, w111) -> (w113:string)
            n46 = call <vilib>:"Create Client.vi"("error in"=w107, "Server Certificate File (.crt)"=w112, "address"=w113) -> ("error out"=w104:errorcluster, "gRPC ID Out"=w102:T52)  [unwired: 7 in]
            n47 = in-place {
              in-place-border: w104 -> [w130]
              in-place-border: [w132] -> w119
              in-place-border: w115 -> [w126]
              in-place-border: w103 -> [w125]
              in-place-border: w114 -> [w124]
              in-place-border: w100 -> [w123]
              in-place-border: w102 -> [w122]
              n48 = in-place-dvr #3(w120) -> (w131:T60, w129:errorcluster)
              n49 = Merge Errors(w130, w129) -> (w128:errorcluster)
              n50 = in-place {
                in-place-border: w128 -> [w137]
                in-place-border: [w137] -> w132
                in-place-border: w125 -> [w136]
                in-place-border: w124 -> [w135]
                in-place-border: w123 -> [w134]
                in-place-border: w122 -> [w133]
                n51 = in-place-map #4(w131, w126) -> (w138:T61)  [unwired: 1 in, 1 out]
                n52 = Bundle By Name(cluster=w138, "gRPC ID"=w133, "grpc_port"=w136, "pid"=w135, "Loader Type"=w134) -> (w140:T61)
                n53 = in-place-map #4(w140, LVMapReplaceAction."Add or Modify Entry" ("action")) -> (w127:T60)  [unwired: 2 out]
              }
              n54 = in-place-dvr #3(w127) -> (w118:errorcluster)  [unwired: 1 out]
            }
            n55 = Merge Errors(w119, w118) -> (w117:errorcluster)
          }
          frame Error {
          }
        }
        n56 = call "Set Manager RegisterPluginLoader Response.vi"("Message Data"=T3 {"void"=""}, "gRPCid in"=w98) -> ("error out"=w96:errorcluster)  [unwired: 9 in]
        n57 = Merge Errors(w91, w96) -> (w99:errorcluster)
      }
      event User Event {
        # "Mark the plugin as ready for removal.  VI Reference will be closed during next timeout to provide plugin time to fully shutdown."
        n58 = event-data() -> ("gRPCid"=w153:T52)  [unwired: 1 in]
        n59 = call "Get Manager UnregisterPlugin Request.vi"("gRPCid"=w153) -> ("error out"=w149:errorcluster, "Message Data"=w146:T62, "gRPCid out"=w152:T52)  [unwired: 8 in]
        n60 = case shown="No Error" w149 {
          selector: w149 -> [w165 w187]
          tunnel: w146 -> [w167 _]
          tunnel: w155 -> [w163 w188]
          tunnel: [w163 w188] -> w154
          tunnel: [w158 w187] -> w148
          frame No Error {
            # "Could add error if plugin not found (should never happen)"
            # "Ignore errors from FIFO destroy.  This is expected if other plugins have already shutdown."
            n61 = Unbundle By Name(w167) -> ("plugin_name"=w157:string)
            n62 = Unbundle By Name(w163) -> ("Plugin Map DVR"=w162:refnum<data-value>)
            n63 = Unbundle By Name(w167) -> ("unregister_channels"=w166:string[])
            n64 = call "Get Plugin Map.vi"("error in (no error)"=w165, "CIFPluginManager in"=w163) -> ("error out"=w161:errorcluster, "Plugin Map"=w164:T54)  [unwired: 8 in]
            n65 = for {
              tunnel: w166 -> [w181] mode=indexing
              tunnel: w164 -> [w176]
              # "Connect to plugin and remove FIFO instance"
              n66 = Match Pattern(string=w181, regular expression="/") -> (before substring=w177:string)  [unwired: 1 in, 3 out]
              n67 = Look In Map(map=w176, key=w177) -> (key not found?=w179:bool, value=w178:T55)  [unwired: 1 in]
              n68 = case shown="False" w179 {
                tunnel: w178 -> [w186 _]
                tunnel: w181 -> [w184 _]
                tunnel: w177 -> [_ _]
                tunnel: [w183 _] -> _
                frame False {
                  n69 = Unbundle By Name(w186) -> ("gRPC ID"=w185:T52)
                  n70 = call <vilib>:"Destroy FIFO Instance.vi"("timeout (ms)"=300, "publisher_instance_name"=w184, "gRPC ID"=w185) -> ("error out"=w183:errorcluster)  [unwired: 7 in, 1 out]
                }
                frame True {
                }
              }
            }
            n71 = in-place {
              in-place-border: [w171] -> w160
              in-place-border: w157 -> [w168]
              n72 = in-place-dvr #5(w162) -> (w170:T54, w171:errorcluster)
              n73 = in-place {
                n74 = in-place-map #6(w170, w168) -> (w174:T55)  [unwired: 1 in, 1 out]
                n75 = Bundle By Name(cluster=w174, "Ready for removal"=TRUE) -> (w173:T55)
                n76 = in-place-map #6(w173, LVMapReplaceAction."Modify Entry only if found" ("action")) -> (w169:T54)  [unwired: 2 out]
              }
              n77 = in-place-dvr #5(w169) -> (w159:errorcluster)  [unwired: 1 out]
            }
            n78 = Merge Errors(w161, w159, w160) -> (w158:errorcluster)
          }
          frame Error {
          }
        }
        n79 = Unbundle By Name(w146) -> ("plugin_name"=w144:string)
        n80 = Concatenate Strings(w144, " unregistered" ("message")) -> (w145:string)
        n81 = call <vilib>:"Write to Syslog.vi"("message"=w145, "CIF Message Type"=Message_Type."Information") -> ()  [unwired: 9 in, 1 out]
        n82 = call "Set Manager UnregisterPlugin Response.vi"("Message Data"=T5 {"void"=""}, "gRPCid in"=w152) -> ("error out"=w151:errorcluster)  [unwired: 9 in]
        n83 = Merge Errors(w148, w151) -> (w156:errorcluster)
      }
      event User Event {
        # "Mark the plugin as ready for removal.  VI Reference will be closed during next timeout to provide plugin time to fully shutdown."
        n84 = event-data() -> ("gRPCid"=w199:T52)  [unwired: 1 in]
        n85 = call "Get Manager UnregisterPluginLoader Request.vi"("gRPCid"=w199) -> ("error out"=w196:errorcluster, "Message Data"=w193:T63, "gRPCid out"=w198:T52)  [unwired: 8 in]
        n86 = case shown="No Error" w196 {
          selector: w196 -> [w203 w219]
          tunnel: w193 -> [w210 _]
          tunnel: w201 -> [w209 w220]
          tunnel: [w209 w220] -> w200
          tunnel: [w205 w219] -> w195
          frame No Error {
            # "Could add error if loader not found (should never happen)"
            n87 = Unbundle By Name(w209) -> ("Loader Map DVR"=w208:refnum<data-value>)
            n88 = Unbundle By Name(w210) -> ("loader_name"=w204:string)
            n89 = in-place {
              in-place-border: [w214] -> w207
              in-place-border: w204 -> [w211]
              n90 = in-place-dvr #7(w208) -> (w213:T60, w214:errorcluster)
              n91 = in-place {
                n92 = in-place-map #8(w213, w211) -> (w217:T61)  [unwired: 1 in, 1 out]
                n93 = Bundle By Name(cluster=w217, "Ready for removal"=TRUE) -> (w216:T61)
                n94 = in-place-map #8(w216, LVMapReplaceAction."Modify Entry only if found" ("action")) -> (w212:T60)  [unwired: 2 out]
              }
              n95 = in-place-dvr #7(w212) -> (w206:errorcluster)  [unwired: 1 out]
            }
            n96 = Merge Errors(w203, w206, w207) -> (w205:errorcluster)
          }
          frame Error {
          }
        }
        n97 = Unbundle By Name(w193) -> ("loader_name"=w191:string)
        n98 = Concatenate Strings(w191, " loader unregistered" ("message")) -> (w192:string)
        n99 = call <vilib>:"Write to Syslog.vi"("message"=w192, "CIF Message Type"=Message_Type."Information") -> ()  [unwired: 9 in, 1 out]
        n100 = call "Set Manager UnregisterPluginLoader Response.vi"("Message Data"=T6 {"void"=""}, "gRPCid in"=w198) -> ("error out"=w197:errorcluster)  [unwired: 9 in]
        n101 = Merge Errors(w195, w197) -> (w202:errorcluster)
      }
      event User Event {
        # "Mark the plugin as ready for removal.  VI Reference will be closed during next timeout to provide plugin time to fully shutdown."
        n102 = event-data() -> ("gRPCid"=w234:T52)  [unwired: 1 in]
        n103 = call "Get Manager QueryPluginTypes Request.vi"("gRPCid"=w234) -> ("error out"=w228:errorcluster, "Message Data"=w227:T64, "gRPCid out"=w233:T52)  [unwired: 8 in]
        n104 = Unbundle By Name(w227) -> ("reload"=w226:bool)
        n105 = case shown="True" w226 {
          tunnel: w229 -> [w237 w241]
          tunnel: [w237 w240] -> w225
          tunnel: [w236 w239] -> w224
          tunnel: w228 -> [w236 w238]
          frame False {
          }
          frame True {
            n106 = call "Trigger Plugin Discovery.vi"("error in (no error)"=w238, "CIFPluginManager in"=w241) -> ("error out"=w239:errorcluster, "CIFPluginManager out"=w240:refnum<class "CIFPluginManager.lvclass">)  [unwired: 8 in]
          }
        }
        n107 = call "Get Discovered Plugin Map.vi"("error in (no error)"=w224, "CIFPluginManager in"=w225) -> ("error out"=w222:errorcluster, "Discovered Plugins"=w223:T65)  [unwired: 8 in]
        n108 = for {
          tunnel: w223 -> [w244] mode=indexing
          tunnel: [w242] -> w231 mode=concatenating
          n109 = Unbundle By Name(w244) -> ("Discovered Plugins"=w243:T66[])
          n110 = for {
            tunnel: w243 -> [w258] mode=indexing
            tunnel: [w252] -> w242 mode=indexing
            n111 = Unbundle By Name(w258) -> ("Plugin Type"=w253:string, "Version.Major"=w254:i32, "Version.Minor"=w255:i32, "Version.Fix"=w256:i32, "Plugin Metadata.Description"=w251:string, "Plugin Metadata.History"=w250:string, "Plugin Metadata.Author"=w249:string, "Relative Path"=w245:string[])
            n112 = To Unsigned Long Integer(number=w254) -> (unsigned 32bit integer=w246:u32)
            n113 = To Unsigned Long Integer(number=w255) -> (unsigned 32bit integer=w247:u32)
            n114 = To Unsigned Long Integer(number=w256) -> (unsigned 32bit integer=w248:u32)
            n115 = Bundle By Name(cluster=T8 {"plugin_type"="", "plugin_version"={"major"=0, "minor"=0, "fix"=0}, "plugin_metadata"={"description"="", "history"="", "author"=""}, "relative_path"=[]} ("cif_manager_PluginType"), "plugin_type"=w253, "plugin_version.major"=w246, "plugin_version.minor"=w247, "plugin_version.fix"=w248, "plugin_metadata.description"=w251, "plugin_metadata.history"=w250, "plugin_metadata.author"=w249, "relative_path"=w245) -> (w252:T8)
          }
        }
        n116 = Bundle By Name(cluster=T7 {"plugin_types"=[]} ("Message Data"), "plugin_types"=w231) -> (w230:T7)
        n117 = call "Set Manager QueryPluginTypes Response.vi"("Message Data"=w230, "gRPCid in"=w233) -> ("error out"=w232:errorcluster)  [unwired: 9 in]
        n118 = Merge Errors(w222, w232) -> (w235:errorcluster)
      }
      event User Event {
        # "Query the channels of all plugins, filter and return the found channels"
        n119 = event-data() -> ("gRPCid"=w274:T52)  [unwired: 1 in]
        n120 = call "Get Manager QueryAllChannels Request.vi"("gRPCid"=w274) -> ("Message Data"=w271:T68, "gRPCid out"=w275:T52)  [unwired: 8 in, 1 out]
        n121 = call "Get Plugin Map.vi"("CIFPluginManager in"=w263) -> ("error out"=w261:errorcluster, "Plugin Map"=w262:T54)  [unwired: 9 in]
        n122 = Unbundle By Name(w271) -> ("channel_filter.name_regex"=w270:string, "channel_filter.direction"=w269:T14, "channel_filter.direction_filter"=w268:bool, "channel_filter.type_regex"=w267:string, "channel_filter.forced"=w266:bool, "channel_filter.forced_filter"=w265:bool)
        n123 = for {
          tunnel: w262 -> [w532] mode=indexing
          tunnel: [w531] -> w272 mode=concatenating
          n124 = Unbundle By Name(w532) -> ("Plugin Management Data.channels.channels"=w531:T13[])
        }
        n125 = for {
          tunnel: w272 -> [w296] mode=indexing
          tunnel: [w296] -> w264 mode=indexing if=w277
          tunnel: w270 -> [w294]
          tunnel: w269 -> [w288]
          tunnel: w268 -> [w284]
          tunnel: w267 -> [w292]
          tunnel: w266 -> [w286]
          tunnel: w265 -> [w283]
          n126 = Unbundle By Name(w296) -> ("name"=w295:string, "type"=w293:string, "direction"=w289:T14, "forced"=w287:bool)
          n127 = Equal?(x=w289, y=w288) -> (x = y?=w285:bool)
          n128 = Equal?(x=w287, y=w286) -> (x = y?=w282:bool)
          n129 = Compound Arithmetic op=OR(w285, invert w284) -> (w279:bool)
          n130 = Compound Arithmetic op=OR(w282, invert w283) -> (w278:bool)
          n131 = xnode "Match Regular Expression"("input string"=w295, "regular expression"=w294) -> ("offset past match"=w291:i32)  [unwired: 4 in, 4 out]
          n132 = xnode "Match Regular Expression"("input string"=w293, "regular expression"=w292) -> ("offset past match"=w290:i32)  [unwired: 4 in, 4 out]
          n133 = Greater Or Equal To 0?(x=w291) -> (x >= 0?=w281:bool)
          n134 = Greater Or Equal To 0?(x=w290) -> (x >= 0?=w280:bool)
          n135 = Compound Arithmetic op=AND(w281, w280, w279, w278) -> (w277:bool)
        }
        n136 = Bundle By Name(cluster=T11 {"channels"={"channels"=[]}} ("Message Data"), "channels.channels"=w264) -> (w259:T11)
        n137 = call "Set Manager QueryAllChannels Response.vi"("Message Data"=w259, "gRPCid in"=w275) -> ("error out"=w273:errorcluster)  [unwired: 9 in]
        n138 = Merge Errors(w261, w273) -> (w276:errorcluster)
      }
      event User Event {
        # "Abort all plugins.  Try to stop the plugins via gRPC command, set the unloading flag and set the timestamp for the timeout/abort."
        n139 = event-data() -> ("gRPCid"=w542:T52)  [unwired: 1 in]
        n140 = Unbundle By Name(w536) -> ("Teardown"=w535:refnum<user-event>)
        n141 = call "Get Manager Destroy Request.vi"("gRPCid"=w542) -> ("error out"=w537:errorcluster, "gRPCid out"=w541:T52)  [unwired: 8 in, 1 out]
        n142 = Generate User Event(user event=w535, event data cluster=TRUE ("event data")) -> (error out=w533:errorcluster)  [unwired: 2 in, 1 out]
        n143 = call "Set Manager Destroy Response.vi"("Message Data"=T5 {"void"=""}, "gRPCid in"=w541) -> ("error out"=w540:errorcluster)  [unwired: 9 in]
        n144 = Merge Errors(w533, w537, w540) -> (w543:errorcluster)
      }
      event User Event {
        n145 = event-data() -> ("gRPCid"=w552:T52)  [unwired: 1 in]
        n146 = call "Get Manager Ping Request.vi"("gRPCid"=w552) -> ("error out"=w550:errorcluster, "gRPCid out"=w551:T52)  [unwired: 8 in, 1 out]
        n147 = call "Create Error Message.vi"("error in (no error)"=w550) -> ("Error Message"=w545:T70)  [unwired: 3 in]
        n148 = Bundle By Name(cluster=T16 {"status"={"code"=0, "message"=""}} ("Message Data"), "status"=w545) -> (w544:T16)
        n149 = call "Set Manager Ping Response.vi"("Message Data"=w544, "gRPCid in"=w551) -> ("error out"=w549:errorcluster)  [unwired: 9 in]
        n150 = Merge Errors(w550, w549) -> (w548:errorcluster)
      }
      event User Event {
        n151 = event-data() -> ("gRPCid"=w565:T52)  [unwired: 1 in]
        n152 = call "Get Manager QueryErrors Request.vi"("gRPCid"=w565) -> ("error out"=w561:errorcluster, "Message Data"=w560:T71, "gRPCid out"=w564:T52)  [unwired: 8 in]
        n153 = Unbundle By Name(w560) -> ("query_settings.query_all"=w559:bool)
        n154 = call "Get Errors.vi"("error in (no error)"=w561, "Parse All"=w559, "Plugin Manager in"=w562) -> ("error out"=w557:errorcluster, "Errors"=w556:T73[], "Plugin Manager out"=w558:refnum<class "CIFPluginManager.lvclass">)  [unwired: 6 in]
        n155 = for {
          tunnel: w556 -> [w575] mode=indexing
          tunnel: [w567] -> w555 mode=indexing
          n156 = Unbundle By Name(w575) -> ("error"=w573:bool, "code"=w572:i32, "Plugin"=w571:string, "Time"=w570:string, "Message"=w569:string, "Location"=w568:string)
          n157 = Bundle By Name(cluster=T20 {"error_status"=FALSE, "error_code"=0, "plugin"="", "time"="", "message"="", "location"=""} ("cif_manager_ErrorInfo"), "error_status"=w573, "error_code"=w572, "plugin"=w571, "time"=w570, "message"=w569, "location"=w568) -> (w567:T20)
        }
        n158 = Bundle By Name(cluster=T18 {"error_info_list"={"error_info"=[]}} ("Message Data"), "error_info_list.error_info"=w555) -> (w554:T18)
        n159 = call "Set Manager QueryErrors Response.vi"("Message Data"=w554, "gRPCid in"=w564) -> ("error out"=w563:errorcluster)  [unwired: 9 in]
        n160 = Merge Errors(w557, w563) -> (w566:errorcluster)
      }
      event User Event {
        n161 = event-data() -> ("gRPCid"=w586:T52)  [unwired: 1 in]
        n162 = call "Get Manager QueryConfig Request.vi"("gRPCid"=w586) -> ("error out"=w582:errorcluster, "Message Data"=w585:T74, "gRPCid out"=w587:T52)  [unwired: 8 in]
        n163 = Unbundle By Name(w585) -> ("query_settings.query_all"=w581:bool)
        n164 = call "Get Config Log.vi"("error in (no error)"=w582, "Parse All"=w581, "Plugin Manager in"=w583) -> ("error out"=w579:errorcluster, "Filtered Config Entries"=w578:string, "Plugin Manager out"=w580:refnum<class "CIFPluginManager.lvclass">)  [unwired: 6 in]
        n165 = Bundle By Name(cluster=T21 {"file_data"={"data"=""}} ("Message Data"), "file_data.data"=w578) -> (w576:T21)
        n166 = call "Set Manager QueryConfig Response.vi"("Message Data"=w576, "gRPCid in"=w587) -> ("error out"=w584:errorcluster)  [unwired: 9 in]
        n167 = Merge Errors(w579, w584) -> (w588:errorcluster)
      }
      event User Event {
        n168 = event-data() -> ("gRPCid"=w600:T52)  [unwired: 1 in]
        n169 = call "Get Manager QueryInfo Request.vi"("gRPCid"=w600) -> ("error out"=w594:errorcluster, "Message Data"=w599:T75, "gRPCid out"=w598:T52)  [unwired: 8 in]
        n170 = Unbundle By Name(w599) -> ("query_settings.query_all"=w595:bool)
        n171 = call "Get Info Log.vi"("error in (no error)"=w594, "Parse All"=w595, "Plugin Manager in"=w596) -> ("error out"=w593:errorcluster, "Filtered Info Entries"=w591:string, "Plugin Manager out"=w592:refnum<class "CIFPluginManager.lvclass">)  [unwired: 6 in]
        n172 = Bundle By Name(cluster=T23 {"file_data"={"data"=""}} ("Message Data"), "file_data.data"=w591) -> (w589:T23)
        n173 = call "Set Manager QueryInfo Response.vi"("Message Data"=w589, "gRPCid in"=w598) -> ("error out"=w597:errorcluster)  [unwired: 9 in]
        n174 = Merge Errors(w593, w597) -> (w601:errorcluster)
      }
      event User Event {
        n175 = event-data() -> ("gRPCid"=w611:T52)  [unwired: 1 in]
        n176 = call "Get Manager ResetErrorIndex Request.vi"("gRPCid"=w611) -> ("error out"=w608:errorcluster, "gRPCid out"=w610:T52)  [unwired: 8 in, 1 out]
        n177 = case shown="No Error" w608 {
          selector: w608 -> [w616 w619]
          tunnel: w607 -> [w618 w620]
          tunnel: [w617 w620] -> w606
          tunnel: [w615 w619] -> w605
          frame No Error {
            n178 = call <vilib>:"Get Last Log Info.vi"("error in"=w616, "CIF Message Type"=Message_Type."Error") -> ("error out"=w615:errorcluster, "Log Info"=w613:T76)  [unwired: 8 in]
            n179 = Bundle By Name(cluster=w618, "Error Log Info"=w613) -> (w617:refnum<class "CIFPluginManager.lvclass">)
          }
          frame Error {
          }
        }
        n180 = call "Create Error Message.vi"("error in (no error)"=w605) -> ("Error Message"=w602:T70)  [unwired: 3 in]
        n181 = Bundle By Name(cluster=T24 {"status"={"code"=0, "message"=""}} ("Message Data"), "status"=w602) -> (w603:T24)
        n182 = call "Set Manager ResetErrorIndex Response.vi"("Message Data"=w603, "gRPCid in"=w610) -> ("error out"=w609:errorcluster)  [unwired: 9 in]
        n183 = Merge Errors(w605, w609) -> (w612:errorcluster)
      }
      event User Event {
        n184 = event-data() -> ("gRPCid"=w627:T52)  [unwired: 1 in]
        n185 = call "Get Manager ResetConfigIndex Request.vi"("gRPCid"=w627) -> ("error out"=w626:errorcluster, "gRPCid out"=w625:T52)  [unwired: 8 in, 1 out]
        n186 = case shown="No Error" w626 {
          selector: w626 -> [w634 w638]
          tunnel: w630 -> [w637 w639]
          tunnel: [w636 w639] -> w629
          tunnel: [w633 w638] -> w628
          frame No Error {
            n187 = call <vilib>:"Get Last Log Info.vi"("error in"=w634, "CIF Message Type"=Message_Type."Configuration") -> ("error out"=w633:errorcluster, "Log Info"=w632:T76)  [unwired: 8 in]
            n188 = Bundle By Name(cluster=w637, "Config Log Info"=w632) -> (w636:refnum<class "CIFPluginManager.lvclass">)
          }
          frame Error {
          }
        }
        n189 = call "Create Error Message.vi"("error in (no error)"=w628) -> ("Error Message"=w621:T70)  [unwired: 3 in]
        n190 = Bundle By Name(cluster=T25 {"status"={"code"=0, "message"=""}} ("Message Data"), "status"=w621) -> (w623:T25)
        n191 = call "Set Manager ResetConfigIndex Response.vi"("Message Data"=w623, "gRPCid in"=w625) -> ("error out"=w624:errorcluster)  [unwired: 9 in]
        n192 = Merge Errors(w628, w624) -> (w631:errorcluster)
      }
      event User Event {
        n193 = event-data() -> ("gRPCid"=w649:T52)  [unwired: 1 in]
        n194 = call "Get Manager ResetInfoIndex Request.vi"("gRPCid"=w649) -> ("error out"=w645:errorcluster, "gRPCid out"=w647:T52)  [unwired: 8 in, 1 out]
        n195 = case shown="No Error" w645 {
          selector: w645 -> [w653 w657]
          tunnel: w646 -> [w656 w658]
          tunnel: [w655 w658] -> w644
          tunnel: [w652 w657] -> w641
          frame No Error {
            n196 = call <vilib>:"Get Last Log Info.vi"("error in"=w653, "CIF Message Type"=Message_Type."Information") -> ("error out"=w652:errorcluster, "Log Info"=w651:T76)  [unwired: 8 in]
            n197 = Bundle By Name(cluster=w656, "Info Log Info"=w651) -> (w655:refnum<class "CIFPluginManager.lvclass">)
          }
          frame Error {
          }
        }
        n198 = call "Create Error Message.vi"("error in (no error)"=w641) -> ("Error Message"=w642:T70)  [unwired: 3 in]
        n199 = Bundle By Name(cluster=T26 {"status"={"code"=0, "message"=""}} ("Message Data"), "status"=w642) -> (w640:T26)
        n200 = call "Set Manager ResetInfoIndex Response.vi"("Message Data"=w640, "gRPCid in"=w647) -> ("error out"=w648:errorcluster)  [unwired: 9 in]
        n201 = Merge Errors(w641, w648) -> (w650:errorcluster)
      }
      event User Event {
        n202 = event-data() -> ("gRPCid"=w668:T52)  [unwired: 1 in]
        n203 = call "Get Manager QueryPluginInfo Request.vi"("gRPCid"=w668) -> ("error out"=w661:errorcluster, "gRPCid out"=w667:T52)  [unwired: 8 in, 1 out]
        n204 = call "Get Plugin Map.vi"("error in (no error)"=w661, "CIFPluginManager in"=w663) -> ("error out"=w660:errorcluster, "Plugin Map"=w662:T54)  [unwired: 8 in]
        n205 = for {
          tunnel: w662 -> [w682] mode=indexing
          tunnel: [w677] -> w665 mode=indexing
          n206 = Unbundle By Name(w682) -> ("Plugin Management Data.status"=w673:T30, "Unique Name"=w680:string, "Plugin Management Data.Plugin Type"=w679:string, "Plugin Management Data.gRPC Port"=w678:i32, "Plugin Management Data.Version.Major"=w674:i32, "Plugin Management Data.Version.Minor"=w675:i32, "Plugin Management Data.Version.Fix"=w676:i32)
          n207 = To Unsigned Long Integer(number=w674) -> (unsigned 32bit integer=w672:u32)
          n208 = To Unsigned Long Integer(number=w675) -> (unsigned 32bit integer=w671:u32)
          n209 = To Unsigned Long Integer(number=w676) -> (unsigned 32bit integer=w670:u32)
          n210 = Bundle By Name(cluster=T29 {"plugin_name"="", "plugin_type"="", "grpc_port"=0, "plugin_version"={"major"=0, "minor"=0, "fix"=0}, "status"={"state"=enum."PLUGINSTATE_UNKNOWN", "timing_statistics"={"period"={"max"=0, "min"=0, "avg"=0.0}, "wake_error"={"max"=0, "min"=0, "avg"=0.0}, "execute"={"max"=0, "min"=0, "avg"=0.0}, "housekeep"={"max"=0, "min"=0, "avg"=0.0}, "idle"={"max"=0, "min"=0, "avg"=0.0}, "cleanup"={"max"=0, "min"=0, "avg"=0.0}, "custom_1"={"max"=0, "min"=0, "avg"=0.0}, "custom_2"={"max"=0, "min"=0, "avg"=0.0}}, "fifo_statistics"={"from_t0"={"max"=0, "min"=0, "avg"=0.0}, "from_previous_plugin"={"max"=0, "min"=0, "avg"=0.0}, "output_error"={"max"=0, "min"=0, "avg"=0.0}}, "error"={"status"=FALSE, "code"=0}, "monitor_doubles"={"double_1"=0.0, "double_2"=0.0, "double_3"=0.0, "double_4"=0.0}, "monitor_u64s"={"u64_1"=0, "u64_2"=0, "u64_3"=0, "u64_4"=0}, "monitor_i64s"={"i64_1"=0, "i64_2"=0, "i64_3"=0, "i64_4"=0}}, "loader_info"={"loader_type"=enum."LOADERTYPE_UNKNOWN", "loader_name"=""}} ("cif_manager_PluginInfo"), "status"=w673, "plugin_name"=w680, "plugin_type"=w679, "grpc_port"=w678, "plugin_version.major"=w672, "plugin_version.minor"=w671, "plugin_version.fix"=w670) -> (w677:T29)
        }
        n211 = Bundle By Name(cluster=T27 {"plugin_info_array"={"plugin_info"=[]}} ("Message Data"), "plugin_info_array.plugin_info"=w665) -> (w664:T27)
        n212 = call "Set Manager QueryPluginInfo Response.vi"("Message Data"=w664, "gRPCid in"=w667) -> ("error out"=w666:errorcluster)  [unwired: 9 in]
        n213 = Merge Errors(w660, w666) -> (w669:errorcluster)
      }
      event User Event {
        # "Don't log query error to main log, only pass to gRPC client."
        n214 = event-data() -> ("gRPCid"=w711:T52)  [unwired: 1 in]
        n215 = call "Get Manager QueryPlugin Request.vi"("gRPCid"=w711) -> ("error out"=w690:errorcluster, "Message Data"=w706:T77, "gRPCid out"=w710:T52)  [unwired: 8 in]
        n216 = Unbundle By Name(w706) -> ("plugin_name"=w697:string)
        n217 = call "Get Plugin Map.vi"("error in (no error)"=w690, "CIFPluginManager in"=w692) -> ("error out"=w689:errorcluster, "Plugin Map"=w691:T54)  [unwired: 8 in]
        n218 = Look In Map(map=w691, key=w697) -> (key not found?=w696:bool, value=w705:T55)  [unwired: 1 in]
        n219 = call <vilib>:"Add Error.vi"("error in (no error)"=w689, "String to Append"=w697, "Error"=Errors."Plugin Not Found", "Insert Error"=w696) -> ("error out"=w698:errorcluster)  [unwired: 7 in]
        n220 = Unbundle By Name(w705) -> ("Loader Type"=w687:T56, "Loader"=w688:string, "status"=w684:T30, "Unique Name"=w685:string, "Plugin Type"=w708:string, "gRPC Port"=w707:i32, "Version.Major"=w704:i32, "Version.Minor"=w702:i32, "Version.Fix"=w703:i32)
        n221 = call "Create Error Message.vi"("error in (no error)"=w698) -> ("Error Message"=w701:T70)  [unwired: 3 in]
        n222 = To Unsigned Long Integer(number=w704) -> (unsigned 32bit integer=w695:u32)
        n223 = To Unsigned Long Integer(number=w702) -> (unsigned 32bit integer=w694:u32)
        n224 = To Unsigned Long Integer(number=w703) -> (unsigned 32bit integer=w693:u32)
        n225 = call "Convert Loader Type to gRPC Type.vi"("Loader Type"=w687) -> ("Loader Type"=w686:T40)  [unwired: 10 in]
        n226 = Bundle By Name(cluster=T41 {"plugin_info"={"plugin_name"="", "plugin_type"="", "grpc_port"=0, "plugin_version"={"major"=0, "minor"=0, "fix"=0}, "status"={"state"=enum."PLUGINSTATE_UNKNOWN", "timing_statistics"={"period"={"max"=0, "min"=0, "avg"=0.0}, "wake_error"={"max"=0, "min"=0, "avg"=0.0}, "execute"={"max"=0, "min"=0, "avg"=0.0}, "housekeep"={"max"=0, "min"=0, "avg"=0.0}, "idle"={"max"=0, "min"=0, "avg"=0.0}, "cleanup"={"max"=0, "min"=0, "avg"=0.0}, "custom_1"={"max"=0, "min"=0, "avg"=0.0}, "custom_2"={"max"=0, "min"=0, "avg"=0.0}}, "fifo_statistics"={"from_t0"={"max"=0, "min"=0, "avg"=0.0}, "from_previous_plugin"={"max"=0, "min"=0, "avg"=0.0}, "output_error"={"max"=0, "min"=0, "avg"=0.0}}, "error"={"status"=FALSE, "code"=0}, "monitor_doubles"={"double_1"=0.0, "double_2"=0.0, "double_3"=0.0, "double_4"=0.0}, "monitor_u64s"={"u64_1"=0, "u64_2"=0, "u64_3"=0, "u64_4"=0}, "monitor_i64s"={"i64_1"=0, "i64_2"=0, "i64_3"=0, "i64_4"=0}}, "loader_info"={"loader_type"=enum."LOADERTYPE_UNKNOWN", "loader_name"=""}}, "status"={"code"=0, "message"=""}} ("Message Data"), "plugin_info.loader_info.loader_type"=w686, "plugin_info.loader_info.loader_name"=w688, "plugin_info.status"=w684, "plugin_info.plugin_name"=w685, "plugin_info.plugin_type"=w708, "plugin_info.grpc_port"=w707, "plugin_info.plugin_version.major"=w695, "plugin_info.plugin_version.minor"=w694, "plugin_info.plugin_version.fix"=w693, "status"=w701) -> (w700:T41)
        n227 = call "Set Manager QueryPlugin Response.vi"("Message Data"=w700, "gRPCid in"=w710) -> ("error out"=w709:errorcluster)  [unwired: 9 in]
        n228 = Merge Errors(w689, w709) -> (w712:errorcluster)
      }
      event User Event {
        n229 = event-data() -> ("gRPCid"=w720:T52)  [unwired: 1 in]
        n230 = call "Get Manager QueryClockStatus Request.vi"("gRPCid"=w720) -> ("error out"=w716:errorcluster, "gRPCid out"=w722:T52)  [unwired: 8 in, 1 out]
        n231 = call "Get Clock History Map.vi"("error in (no error)"=w716, "CIFPluginManager in"=w718) -> ("error out"=w715:errorcluster, "Clock History Map"=w717:T78)  [unwired: 8 in]
        n232 = call <vilib>:"Clock Map to Clock Array.vi"("error in (no error)"=w715, "Clock History Map in"=w717) -> ("error out"=w724:errorcluster, "Clock Conversion Array"=w723:T80[], "Clock History Map out"=w719:T78)  [unwired: 7 in]
        n233 = for {
          tunnel: w723 -> [w740] mode=indexing
          tunnel: [w733] -> w725 mode=indexing
          tunnel: w719 -> [w731]
          n234 = Unbundle By Name(w740) -> ("ClockID"=w730:u8, "Last Reset"=w734:i64, "Offset Pair.System Time"=w735:i64, "Offset Pair.External Time"=w736:i64, "Slope"=w737:dbl, "Name"=w738:string)
          n235 = To Unsigned Long Integer(number=w730) -> (unsigned 32bit integer=w739:u32)
          n236 = call <vilib>:"Calculate Error.vi"("ClockID"=w730, "Clock History Map in"=w731) -> ("Error Statistics (ns)"=w729:T81)  [unwired: 8 in, 1 out]
          n237 = Unbundle By Name(w729) -> ("mean"=w728:i64, "standard deviation"=w727:i64)
          n238 = Bundle By Name(cluster=T45 {"clock_conversion"={"clock_id"=0, "last_reset"=0, "slope"=0.0, "offset_pair"={"system_time"=0, "external_time"=0}, "clock_name"=""}, "error_mean"=0, "error_std_dev"=0} ("cif_manager_ClockStatus"), "error_mean"=w728, "error_std_dev"=w727, "clock_conversion.clock_id"=w739, "clock_conversion.last_reset"=w734, "clock_conversion.offset_pair.system_time"=w735, "clock_conversion.offset_pair.external_time"=w736, "clock_conversion.slope"=w737, "clock_conversion.clock_name"=w738) -> (w733:T45)
        }
        n239 = Bundle By Name(cluster=T43 {"clock_status_array"={"clocks_status"=[]}} ("Message Data"), "clock_status_array.clocks_status"=w725) -> (w713:T43)
        n240 = call "Set Manager QueryClockStatus Response.vi"("Message Data"=w713, "gRPCid in"=w722) -> ("error out"=w721:errorcluster)  [unwired: 9 in]
        n241 = Merge Errors(w724, w721) -> (w726:errorcluster)
      }
      event User Event {
        # "Could add clock log function"
        n242 = event-data() -> ("gRPCid"=w753:T52)  [unwired: 1 in]
        n243 = call "Get Manager UpdateClock Request.vi"("gRPCid"=w753) -> ("error out"=w750:errorcluster, "Message Data"=w749:T82, "gRPCid out"=w752:T52)  [unwired: 8 in]
        n244 = Unbundle By Name(w748) -> ("Clock History Map DVR"=w747:refnum<data-value>)
        n245 = in-place {
          in-place-border: [w769] -> w746
          in-place-border: w750 -> [w757]
          in-place-border: w749 -> [w768]
          n246 = in-place-dvr #9(w747) -> (w759:T78, w756:errorcluster)
          n247 = Merge Errors(w757, w756) -> (w755:errorcluster)
          n248 = Unbundle By Name(w768) -> ("timestamp_pair.system_time"=w762:i64, "timestamp_pair.external_time"=w761:i64, "reinit"=w764:bool, "clock_id"=w767:u32, "clock_name"=w766:string)
          n249 = Bundle By Name(cluster=T49 {"System Time"=0, "External Time"=0} ("Timestamp Pair"), "System Time"=w762, "External Time"=w761) -> (w760:T49)
          n250 = To Unsigned Byte Integer(number=w767) -> (unsigned 8bit integer=w765:u8)
          n251 = call <vilib>:"Update Clock Map.vi"("Name"=w766, "Reset"=w764, "error in (no error)"=w755, "ClockID"=w765, "Timestamp Pair"=w760, "Clock History Map in"=w759) -> ("error out"=w769:errorcluster, "Clock History Map out"=w758:map{u8, T79})  [unwired: 4 in]
          n252 = in-place-dvr #9(w758) -> (w745:errorcluster)  [unwired: 1 out]
        }
        n253 = Merge Errors(w746, w745) -> (w744:errorcluster)
        n254 = call "Create Error Message.vi"("error in (no error)"=w744) -> ("Error Message"=w743:T70)  [unwired: 3 in]
        n255 = Bundle By Name(cluster=T48 {"status"={"code"=0, "message"=""}} ("Message Data"), "status"=w743) -> (w741:T48)
        n256 = call "Set Manager UpdateClock Response.vi"("Message Data"=w741, "gRPCid in"=w752) -> ("error out"=w751:errorcluster)  [unwired: 9 in]
        n257 = Merge Errors(w744, w751) -> (w754:errorcluster)
      }
      event User Event {
        n258 = event-data() -> ("gRPCid"=w801:T52)  [unwired: 1 in]
        n259 = call "Get Manager CreateOrch Request.vi"("gRPCid"=w801) -> ("error out"=w796:errorcluster, "Message Data"=w795:T83, "gRPCid out"=w800:T52)  [unwired: 8 in]
        n260 = Unbundle By Name(w795) -> ("start_timestamp"=w772:u64, "filename"=w790:string, "default_ip"=w791:string, "orchestration_language"=w786:T84, "create_file"=w785:bool)
        n261 = To Quad Integer(1:w772) -> (0:w770:i64)
        n262 = call <vilib>:"TAI Time to LabVIEW Time.vi"("TAI Time (ns)"=w770) -> ("LabVIEW Time (s)"=w773:timestamp)  [unwired: 4 in]
        n263 = Not Equal To 0?(x=w772) -> (x != 0?=w794:bool)
        n264 = call <vilib>:"Trim Whitespace.vi"("string"=w790) -> ("trimmed string"=w776:string)  [unwired: 1 in]
        n265 = call <vilib>:"Trim Whitespace.vi"("string"=w791) -> ("trimmed string"=w789:string)  [unwired: 1 in]
        n266 = Format Date/Time String(time format string (%c)="%m/%d/%Y %H:%M:%S", seconds (now)=w773, UTC format=TRUE) -> (date/time string=w771:string)
        n267 = call "Get Config Log.vi"("Parse Timestamp"=w771, "error in (no error)"=w796, "Parse All"=w794, "Plugin Manager in"=w798) -> ("error out"=w792:errorcluster, "Filtered Config Entries"=w793:string, "Plugin Manager out"=w797:refnum<class "CIFPluginManager.lvclass">)  [unwired: 5 in]
        n268 = Empty String/Path?(string/path=w789) -> (empty?=w788:bool)
        n269 = Not(x=w788) -> (.not. x?=w787:bool)
        n270 = case shown="\"ORCHESTRATIONLANGUAGE_PYTHON\", Default" w786 {
          tunnel: w793 -> [w815]
          tunnel: w792 -> [w814]
          tunnel: w776 -> [w813]
          tunnel: w789 -> [w812]
          tunnel: w787 -> [w811]
          tunnel: [w810] -> w783
          tunnel: [w809] -> w784
          tunnel: [w808] -> w777
          frame "ORCHESTRATIONLANGUAGE_PYTHON", Default {
            n271 = call "Create Python Orchestration Script.vi"("Override Address"=w811, "error in"=w814, "Default Address"=w812, "Configuration File Name"=w813, "Filtered Config Entries"=w815) -> ("error out"=w810:errorcluster, "Orchestration File Path"=w809:path, "Python Orchestration File"=w808:string)  [unwired: 4 in]
          }
        }
        n272 = case shown="True" w785 {
          tunnel: w777 -> [_ w805]
          tunnel: w784 -> [_ w806]
          tunnel: w783 -> [w803 w807]
          tunnel: [w803 w804] -> w780
          frame False {
          }
          frame True {
            n273 = Write to Text File(file (use dialog)=w806, text=w805, error in=w807) -> (error out=w804:errorcluster)  [unwired: 1 in, 2 out]
          }
        }
        n274 = call "Create Error Message.vi"("error in (no error)"=w780) -> ("Error Message"=w781:T70)  [unwired: 3 in]
        n275 = Bundle By Name(cluster=T50 {"orchestration_script"="", "status"={"code"=0, "message"=""}} ("Message Data"), "status"=w781) -> (w779:T50)
        n276 = Bundle By Name(cluster=w779, "orchestration_script"=w777) -> (w778:T50)
        n277 = call "Set Manager CreateOrch Response.vi"("Message Data"=w778, "gRPCid in"=w800) -> ("error out"=w799:errorcluster)  [unwired: 9 in]
        n278 = Merge Errors(w780, w799) -> (w802:errorcluster)
      }
      event User Event {
        # "Ignore socket closed error"
        # "For faster UI don't wait on loader to respond"
        n279 = event-data() -> ("gRPCid"=w829:T52)  [unwired: 1 in]
        n280 = call "Get Manager DestroyPluginLoader Request.vi"("gRPCid"=w829) -> ("error out"=w823:errorcluster, "Message Data"=w825:T85, "gRPCid out"=w828:T52)  [unwired: 8 in]
        n281 = Unbundle By Name(w825) -> ("loader_name"=w822:string)
        n282 = call "Request Plugin Loader Stop.vi"("error in (no error)"=w823, "Plugin Loader Name"=w822, "CIFPluginManager in"=w824) -> ("error out"=w819:errorcluster, "gRPC ID"=w821:T52)  [unwired: 7 in]
        n283 = call "Destroy Loader.vi"("error in"=w819, "gRPC ID in"=w821) -> ("error out"=w820:errorcluster)  [unwired: 8 in, 1 out]
        n284 = call <vilib>:"Clear Errors.vi"("error in (no error)"=w820, "specific error code to clear (0: all)"=-1014) -> ("error out"=w826:errorcluster)  [unwired: 4 in, 1 out]
        n285 = call "Create Error Message.vi"("error in (no error)"=w819) -> ("Error Message"=w817:T70)  [unwired: 3 in]
        n286 = Bundle By Name(cluster=T51 {"status"={"code"=0, "message"=""}} ("Message Data"), "status"=w817) -> (w816:T51)
        n287 = call "Set Manager DestroyPluginLoader Response.vi"("Message Data"=w816, "gRPCid in"=w828) -> ("error out"=w827:errorcluster)  [unwired: 9 in]
        n288 = Merge Errors(w826, w827) -> (w831:errorcluster)
      }
      event User Event {
        n289 = event-data() -> ()  [unwired: 1 in, 2 out]
        n290 = Unbundle By Name(w833) -> ("Shutdown"=w834:refnum<user-event>)
        n291 = Generate User Event(user event=w834, event data cluster=TRUE ("event data")) -> ()  [unwired: 2 in, 2 out]
      }
    }
    n292 = call <vilib>:"Filter and Log Error.vi"("error In"=w13, "Name"=w9) -> ()  [unwired: 10 in]
  }
  "Plugin Manager out" <- w5
  n293 = Unregister For Events(event registration refnum=w6) -> (error out=→"error out":errorcluster)  [unwired: 1 in]
